vi "Dashboard Main.vi"() -> ()   [LabVIEW 2018]
uses:
  <vilib>/Utility/miscctls.llb/LVRowAndColumnTypeDef.ctl
  <vilib>/event_ctls.llb/eventvkey.ctl
  <vilib>/Utility/xml.llb/Read From XML File(array).vi
  <vilib>/Utility/xml.llb/Write to XML File(string).vi
  <vilib>/Rock Robotics/Network Tables/NT Read Boolean.vi
  <vilib>/Rock Robotics/Network Tables/NT Write Boolean.vi
  <vilib>/Rock Robotics/WPI/Dashboard/WPI_DashboardLogging Global.vi
  <vilib>/vision/NI_Vision_Development_Module.lvlib
panel:
  in  "TCP":refnum<k5>
  in  "Rec Mode":enum32{"Stop", "Record", "Playback"}(radio)
  out "Image Message":string="Timeout in Camera Communications"
  in  "Dashboard Tab":T1(tab)=enum."TeleOp"
  in  "CheckList":i32(listbox)
  in  "Driver Profile":u16(ring) items=["N/A"]
  in  "Camera Name":string(combo)="limelight"
  in  "Camera Settings":T2={"Frame Rate"=20, "Compression"=60, "Size"=1, "DB Camera Config"=FALSE} {"Size" items=["640x480", "320x240", "160x120"]}
  in  "Warning Time (s)":dbl=30.0
  in  "Autonomous Play":u16(ring) items=["N/A"]
  in  "Refresh_Auto_Play_List":bool
  out "Pressure_Leak":bool
  out "Ret_CARGO Right":bool
  out "Ret_HATCH Right":bool
  out "Ret_CARGO Left":bool
  out "Ret_HATCH Left":bool
  out "Ret_CARGO Center":bool
  out "Elevator_Motor_Failure_2":bool
  out "Elevator_Stall":bool
  out "Range_Color_Front-Right":u32(colorbox)
  in  "Right":bool
  in  "Reticule":T3(ring)
  in  "Save":bool
  in  "Up":bool
  in  "Down":bool
  in  "Left":bool
  out "Out_Of_Time":bool caption="Mode_Butterfly"
  out "Match Time(s)":sgl
  out "Intake_In":bool caption="Mode_Butterfly"
  in  "Climb_Safety":bool
  out "Master_Caution":bool caption="Mode_Butterfly"
  out "Climb_Sequence":string
  out "Range_to_Target (R)":i16(slide)=-100 scale=-10.0..-50.0
  out "Range_to_Target (L)":i16(slide)=-100 scale=-50.0..-10.0
  out "Tilt_Interlock":bool
  out "Battery_Critical":bool
  out "Battery_Voltage":dbl(slide) scale=11.0..13.0
  out "COM_Warning":bool
  out "Elevator_Moving":bool caption="Mode_Butterfly"
  out "Range_Color_Back":u32(colorbox)
  out "Range_Color_Front-Left":u32(colorbox)
  out "Range_Color_Right":u32(colorbox)
  out "Range_Color_Left":u32(colorbox)
  out "Hatch_Ship_Light":bool
  out "Hatch_Rocket_1_Light":bool
  out "Hatch_Ground_Light":bool
  out "Hatch_Feeder_Light":bool
  out "Hatch_Rocket_2_Light":bool
  out "Hatch_Rocket_3_Light":bool
  out "Pressure_Visualize":dbl(slide) scale=0.0..120.0
  out "Autopilot":bool caption="Mode_Butterfly"
  in  "Master_Safety_Override_1":bool
  in  "Master_Safety_Override_2":bool
  out "Climb_Light":bool
  out "At Climb_Height":bool caption="Mode_Butterfly"
  out "PTO_Engaged":bool caption="Mode_Butterfly"
  in  "Climb":bool
  out "Mode_Butterfly":bool
  out "Compressor_On":bool
  out "Hatch_Ejection_State":bool caption="Mode_Butterfly"
  out "Elevator_Brake_State":bool
  out "Mode_Shift":bool caption="Mode_Butterfly"
  out "Capture_Cargo":bool caption="Mode_Butterfly"
  out "Capture_Hatch":bool caption="Mode_Butterfly"
  in  "Hatch_Ground":bool
  in  "Hatch_Feeder":bool
  in  "Hatch_Rocket_2":bool
  in  "Hatch_Rocket_1":bool
  in  "Hatch_Ship":bool
  in  "Hatch_Rocket_3":bool
  out "Elevator_Stow_Light":bool
  in  "Elevator_Stow":bool
  out "Cargo_Ground_Light":bool
  out "Cargo_Feeder_Light":bool
  out "Cargo_Ship_Light":bool
  out "Cargo_Rocket_3_Light":bool
  in  "Cargo_Ground":bool
  in  "Cargo_Feeder":bool
  out "Cargo_Rocket_2_Light":bool
  out "Cargo_Rocket_1_Light":bool
  in  "Cargo_Ship":bool
  in  "Cargo_Rocket_1":bool
  in  "Cargo_Rocket_2":bool
  in  "Cargo_Rocket_3":bool
  out "State_Conflict":bool caption="Mode_Butterfly"
  out "Combined Camera Feed":T4(plugin-control)
  out "Elevator_Pos_Visual":dbl(slide) scale=34.5..89.0
  in  "Vision_Target_L_R":bool
  out "Elevator_Goal_Visual":dbl(slide) scale=34.5..89.0
  out "Elevator_Power":dbl(knob) scale=-1.0..1.0
  in  "Climb_Level":u8(slide)=1 scale=0.0..2.0
  out "E1 Warning":bool
  out "E2 Warning":bool
  out "E3 Warning":bool
  out "Elevator_3_Current":dbl format="%.1g"
  out "Elevator_2_Current":dbl format="%.1g"
  out "Elevator_1_Current":dbl format="%.1g"
  out "Slow_Loop":bool
  in  "Elevator_Kf_1":dbl(slide)=0.2 min=0.0 max=1.0 scale=0.0..1.0
  in  "Elevator_Kf_2":dbl(slide)=0.2 min=0.0 max=1.0 scale=0.0..1.0
  in  "Elevator_Kf_3":dbl(slide) min=0.0 max=1.0 scale=0.0..1.0
  in  "Select Auto":string(combo)="Select Autonomous ..."
  out "Camera Perf":string
  in  "Elevator_Kf_Climb":dbl(slide)=0.1 min=0.0 max=1.0 scale=0.0..1.0
  out "Control Loop Time (ms)":u32
  in  "Vacuum_Pump":dbl(slide)=0.6 min=0.0 max=1.0 scale=0.0..1.0
  out "Range_Right":dbl format="%.1g"
  in  "Elevator_Manual":bool
  in  "Drive_Encoder_Reset":bool
  out "Right_Drive_Pos":dbl
  out "Left_Drive_Pos":dbl
  out "Range_Left":dbl format="%.1g"
  out "Range_Front-Left":dbl format="%.1g"
  out "Range_Front-Right":dbl format="%.1g"
  out "Left_Drive_Vel":dbl format="%.1g"
  out "Right_Drive_Vel":dbl format="%.1g"
  out "Elevator_Pos":dbl format="%.1g"
  out "Range_Back":dbl
  out "Tank_Pressure":dbl format="%.1f"
  in  "Super_Test_Mode":bool
  out "Ground_Height":dbl format="%.1g"
  in  "Overclock":bool=TRUE
  in  "Reinit_Stow_Vacuum":bool
  in  "LimeLight_Override":bool
  out "Elevator_Encoder_Malfunction":bool
  out "Elevator_Motor_Failure":bool
  out "Robot_On_Ground":bool=TRUE
  out "Robot_Off_Ground":bool
  out "Check_Limit_Switch":bool
  in  "Tilt_Safety_Override":bool
  in  "Defense_Driving":bool
  out "Combined Error String":string
  out "NT Connection":bool
  out "Mode":T5(ring)=enum."Auto Disabled"
  in  "Test Slider":dbl(slide) scale=0.0..100.0 scale format="%#_3g"
  in  "On/Off":bool caption="Solenoid"
  in  "Test Name":u16(ring) items=["Select the test to run..."]
  in  "Test Tree":string(tree)
  in  "Motor":cluster{"Value":dbl, "Enable":bool} {"Value" scale=-1.0..1.0 scale format="%#_3g"}
  out "Progress":T6 {"Test Progress" scale=0.0..100.0}
  in  "Rev/Fwd":cluster{"Forward":bool, "Reverse":bool}
  in  "Test Ring":u16(ring) items=["Monochrome", "Color"]
  out "Cmd Status":string
  in  "Execute Command":bool
  in  "Command Params":string[][](table)
  in  "Command Selection":i32(listbox)
  out "Tree":string(tree)
  out "Background":bool
  # "Refresh Auto Plays List"
  # "Camera Selection"
  # "Match End Warning (s)"
  # "Camera Settings"
  # "Safe"
  # "89.0"
  # "11"
  # "13"
  # "120"
  # "0"
  # "Valkyrie"
  # "B"
  # "3"
  # "2"
  # "0"
  # "34.5"
  # "Control Loop (ms)"
  # "Elevator Feed Forward Coefficients"
  # "Drive Wheel Velocities (ft/s)"
  # "Manual Elevator Override"
  # "Tilt Interlock Off"
  # "Wide-Cam Override"
  # "Reinit.  Vacuum in Stow"
  # "Super Test Mode"
  # "Elevator Position (in)"
  # "Prox Sensors (in)"
  # "Auto Elevator"
  # "Safe"
  # "Vacuum \nPump Power"
  # "Normal"
  # "Normal"
  # "Safe"
  # "Stage 2"
  # "Stage 3"
  # "Climb"
  # "Ground Height (in)"
  # "Elevator Motor Currents (A)"
  # "On \nGround"
  # "Off\nGround"
  # "E1"
  # "E2"
  # "E3"
  # "Tank Pressure (psi)"
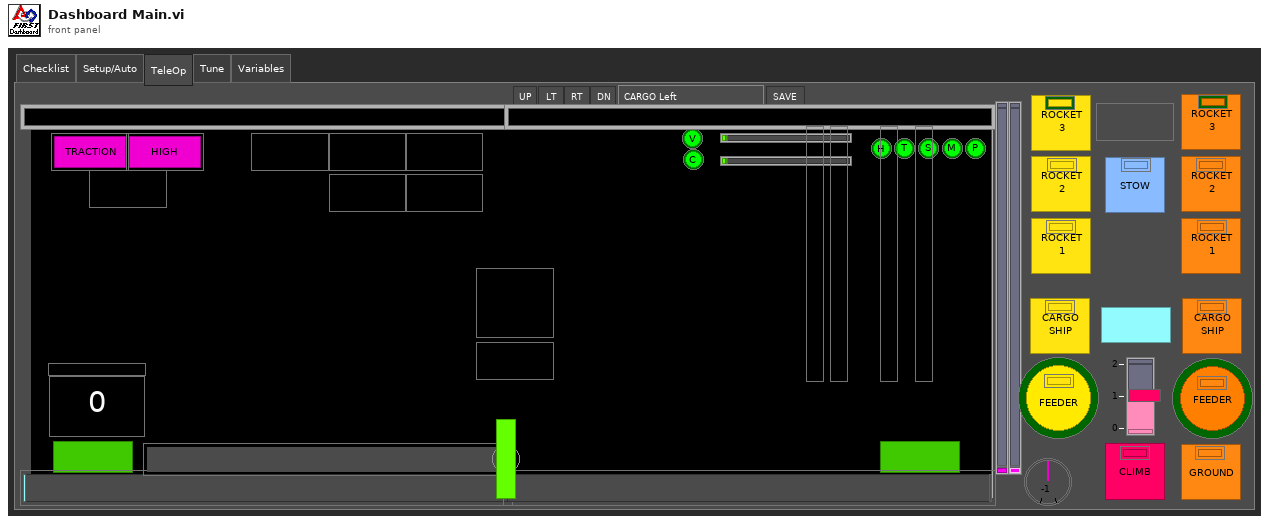
[diagram p1: front panel]
types:
  T1 = enum32{"Checklist", "Setup/Auto", "TeleOp", "Tune", "NT", "Test", "Commands", "Variables"}
  T2 = cluster{"Frame Rate":i32, "Compression":i32, "Size":u16, "DB Camera Config":bool}
  T3 = enum16{"CARGO Left", "CARGO Right", "HATCH Left", "HATCH Right", "CARGO Center"}
  T4 = typedef "IMAQ Image.ctl" = refnum<image>
  T5 = enum8{"Tele-Op Disabled", "Tele-Op Enabled", "Auto Disabled", "Auto Enabled", "Test Disabled", "Test Enabled", "Disconnected", "No Code", "E-Stop"}
  T6 = cluster{"Test Progress":u8, "Test Progress Text":string}
  T7 = cluster{"Save Path":path, "Interval (s)":dbl, "Keep":i32}
  T8 = enum32{"Drive", "Camera", "Basic", "Custom", "Test", "Commands", "Checklist", "Variables"}
  T9 = cluster{"IDs":cluster{"RPC field ID":u16, "Unique ID":u16}, "String":string}
  T10 = typedef "Image Type" = u32
  T11 = cluster{"Camera Name":string, string, "Saved DB Images Info":cluster{"Save Path":path, "Interval (s)":dbl, "Keep":i32}}
  T12 = cluster{"Ret_CARGO Left":refnum<vi>, "Ret_CARGO Right":refnum<vi>, "Ret_HATCH Left":refnum<vi>, "Ret_HATCH Right":refnum<vi>, "Ret_CARGO Center":refnum<vi>}
  T13 = enum32{"Checklist", "-", "TeleOp", "Tune", "NT", "Test", "Commands", "Variables"}
  T14 = cluster{"Error Strings":string, "Disable Counts":cluster{u16, u16}, "Rail Faults":cluster{u16, u16, u16}, "Robot IP":string, "DB Mode":u8, "Event Info":cluster{"Name":string, "Type":u8, "Number":u16, "Replay":u8}}
  T15 = cluster{"Storage":cluster{"Disk Free":u64, "RAM Block":u32, "RAM free":u32}, "CPU Utilization":cluster{"CPU % ISR":sgl, "CPU % Time Crit":sgl, "CPU % Timed Str":sgl, "CPU % High":sgl, "CPU % Above":sgl, "CPU % Normal":sgl, "CPU % Low":sgl}, "CAN":cluster{"% Bus Utilization":sgl, "Bus Off Cnt":u32, "TX_FIFO Full Cnt":u32, "Receive Error Cnt":u8, "Transmit Error Cnt":u8}, "HID":cluster{"HID Outputs":u32, "Rumble Low":u16, "Rumble High":u16}[]}
  T16 = cluster{"Status bits":cluster{"Test Mode":bool, "Autonomous":bool, "Enabled":bool, "Code Start":bool, "Brownout":bool, "Reserved 2":bool, "Reserved 3":bool, "E-Stop":bool}, "Code Trace":cluster{"Disabled":bool, "TeleOp":bool, "Auto":bool, "Test":bool}, "Controller Type":enum16{"unknown", "cRIO", "roboRio"}, "Code?":enum16{"unknown", "noCode", "code"}, "Battery V":dbl}
  T17 = cluster{"Control Bits":cluster{"TestMode":bool, "Autonomous":bool, "Enabled":bool, "FMS Present":bool, bool, bool, bool, "E-Stop":bool}, "Team Station ":u8, "Countdown":sgl, "Joystick Values":cluster{"Axes":dbl[], "Buttons":bool[], "POVs":i16[]}[]}
  T18 = cluster{"Operation":enum16{"Update", "Clear"}, "Color Box":u32}[]
  T19 = typedef "eventvkey.ctl" = enum16{"ASCII", "Enter", "Return", "Shift", "Ctrl", "Alt", "Cmd", "Opt", "Caps", "NumLock", "Clear", "Break", "Up", "Down", "Left", "Right", "Insert", "Delete", "Home", "End", "PageUp", "PageDown", "Escape", "Help", "Pause", "ScrollLock", "F1", "F2", "F3", "F4", "F5", "F6", "F7", "F8", "F9", "F10", "F11", "F12", "F13", "F14", "F15", "F16", "F17", "F18", "F19", "F20", "F21", "F22", "F23", "F24", "Play", "VolumeUp", "VolumeDown", "Mute", "Two Byte Char"}
  T20 = cluster{"Image Size":bool, "Image Type":bool, "Pixel Value":bool, "ROI Information":bool, "Zoom Factor":bool}
  T21 = cluster{"Operation":enum16{"Update", "Clear"}, "Color Box":u32}
  T22 = typedef "LVRowAndColumnTypeDef.ctl" = cluster{"Row":i32, "Column":i32}
  T23 = cluster{"Shift":bool, "Ctrl":bool, "Alt":bool, "Cmd":bool, "Opt":bool}
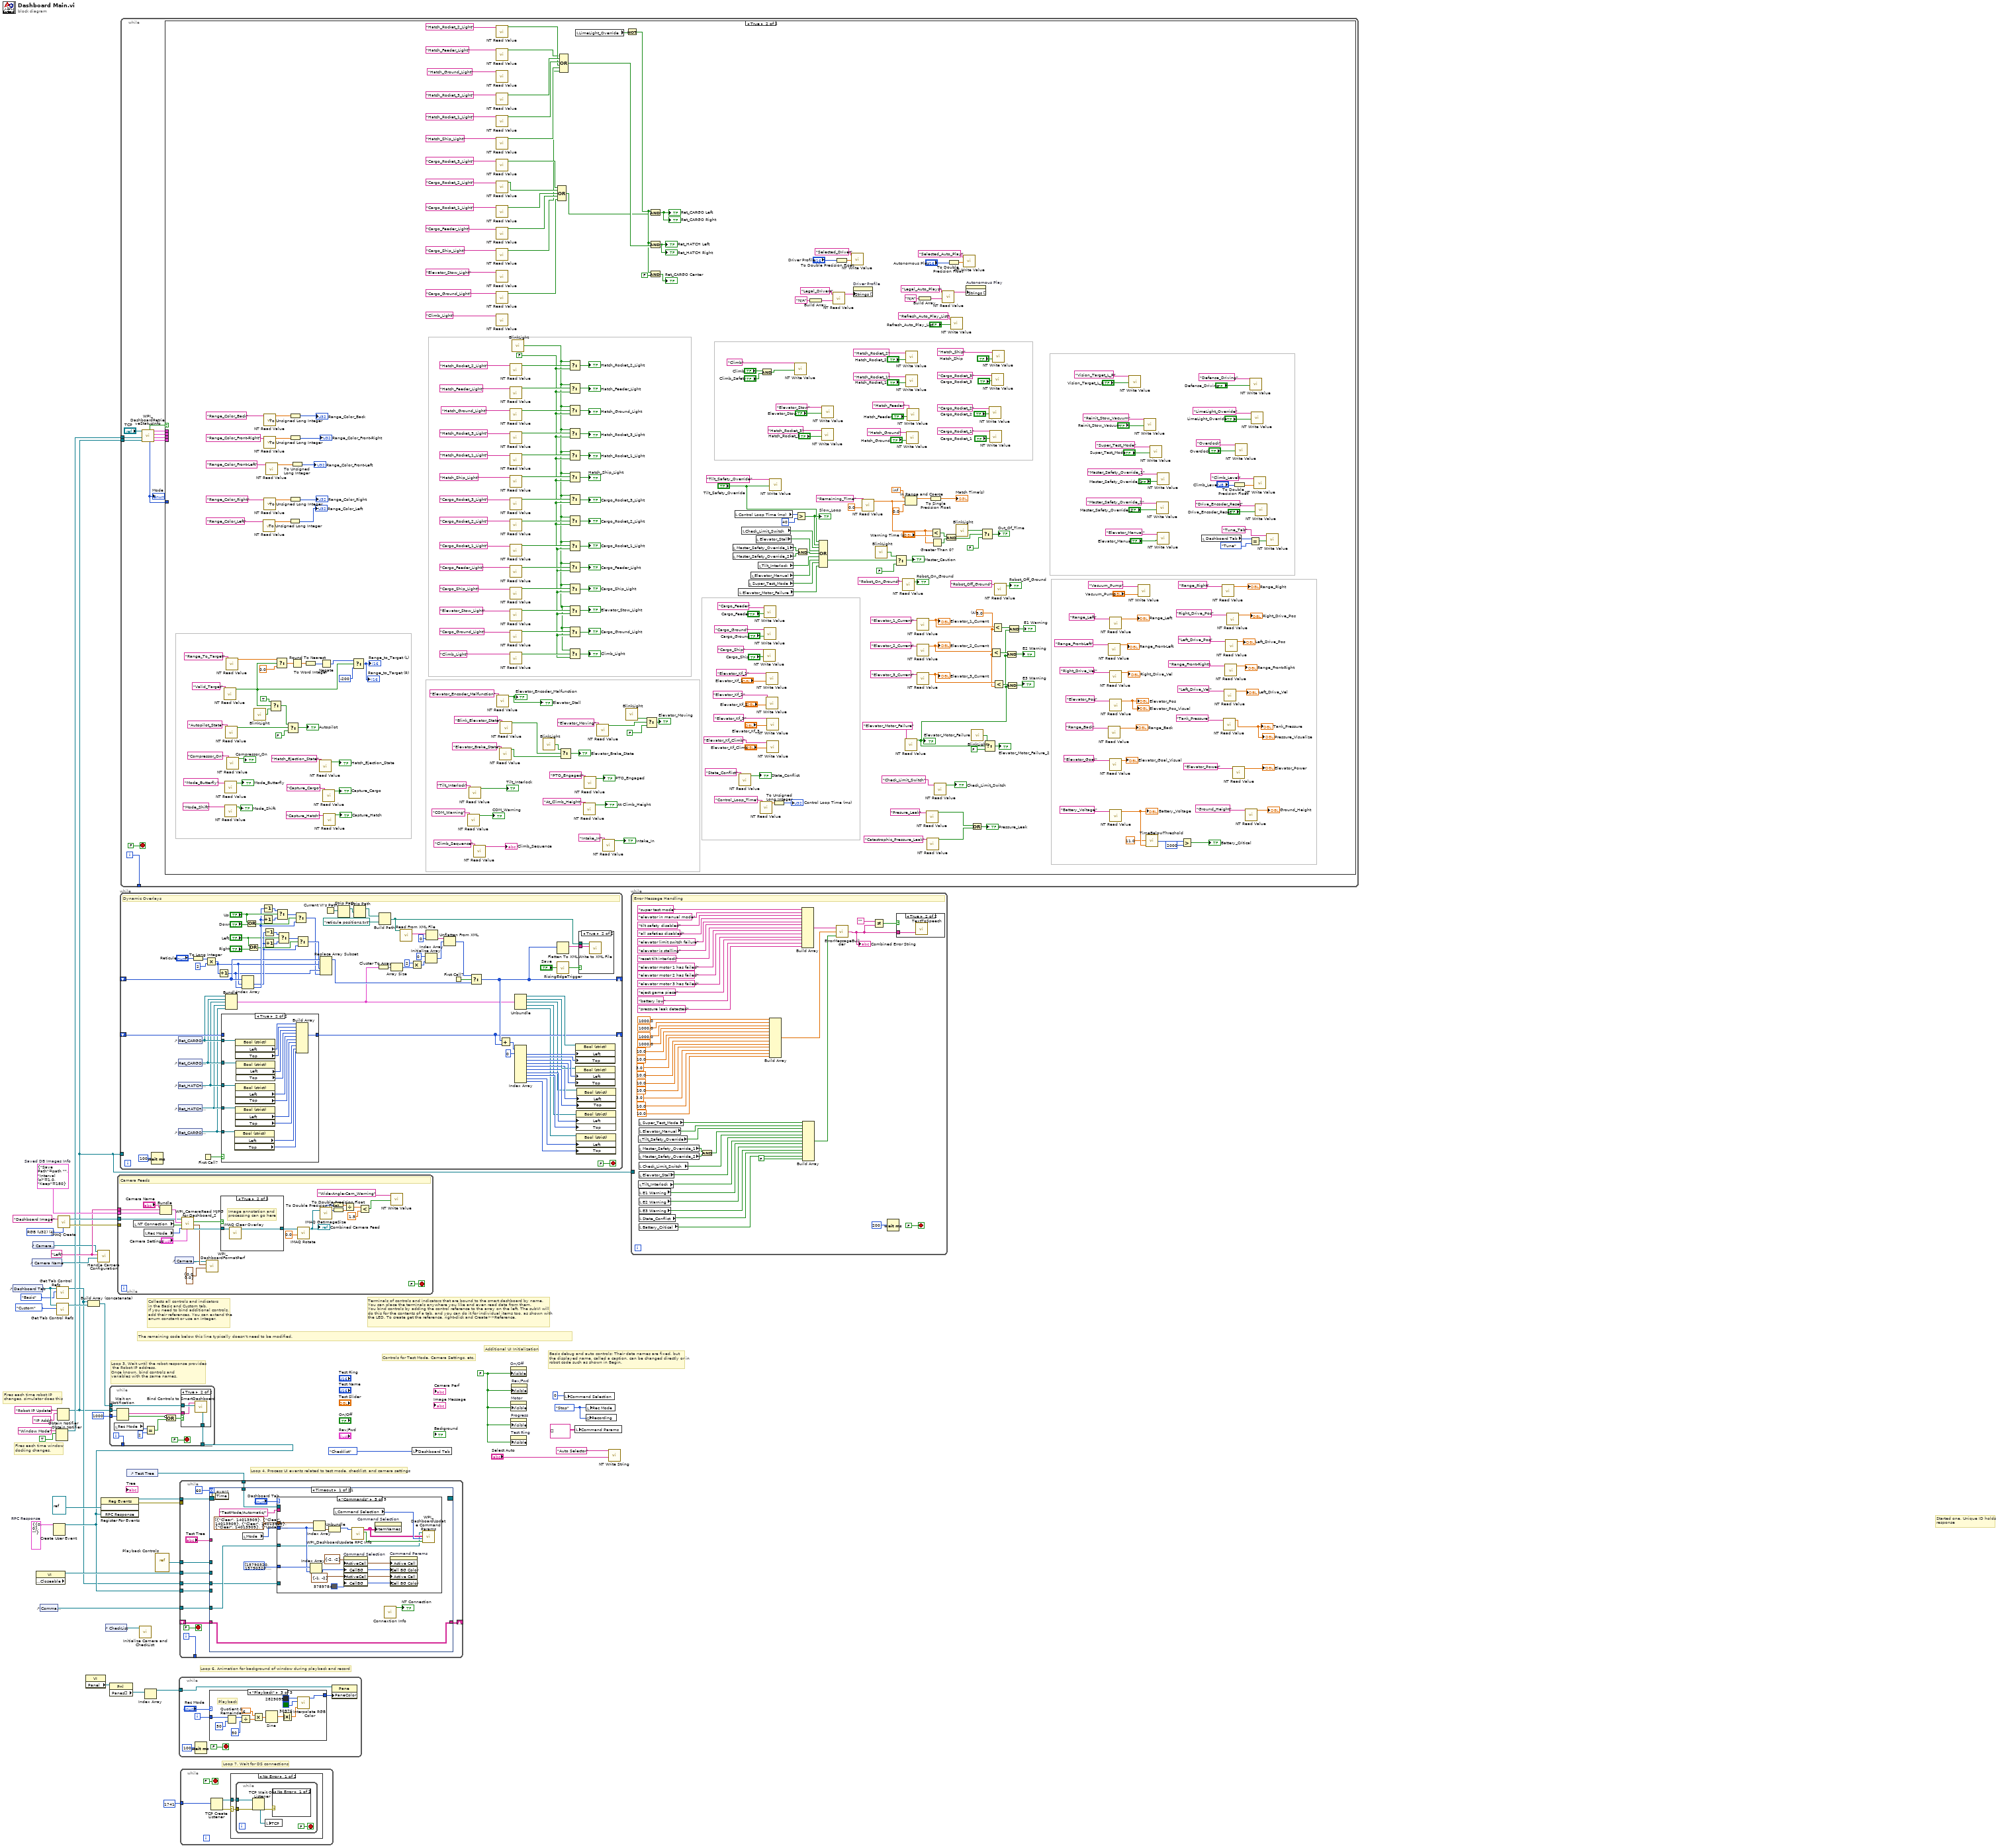
[diagram p0: block diagram]
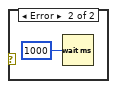
[diagram p5: hidden frame]
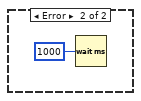
[diagram p6: hidden frame]
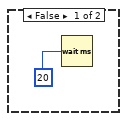
[diagram p7: hidden frame]
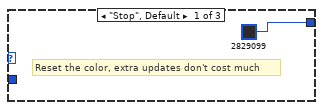
[diagram p8: hidden frame]
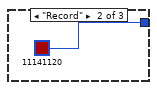
[diagram p9: hidden frame]
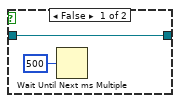
[diagram p11: hidden frame]
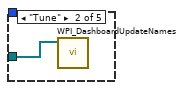
[diagram p13: hidden frame]
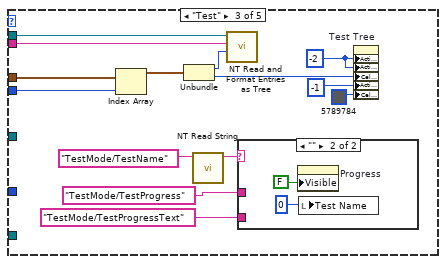
[diagram p14: hidden frame]
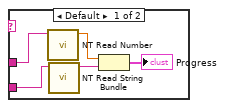
[diagram p15: hidden frame]
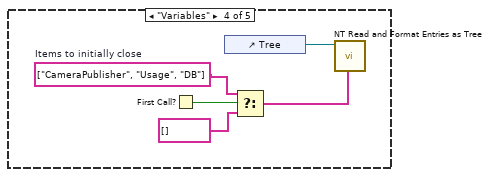
[diagram p16: hidden frame]
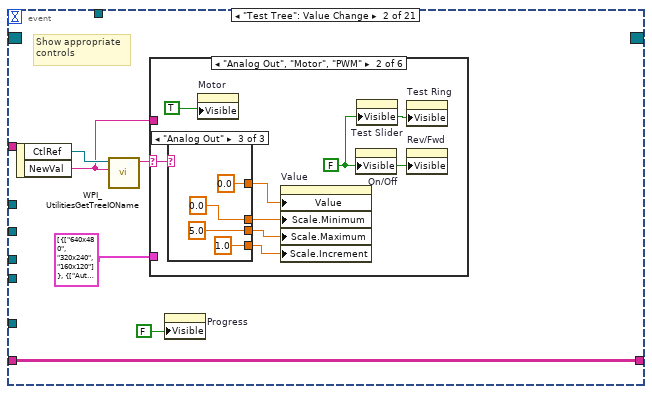
[diagram p17: hidden frame]
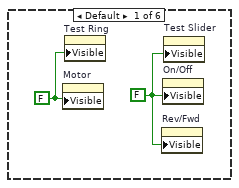
[diagram p18: hidden frame]
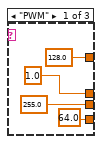
[diagram p19: hidden frame]
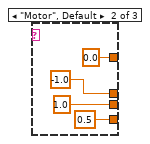
[diagram p20: hidden frame]
diagram:
  w4 = T7 {"Save Path"=path "", "Interval (s)"=1.0, "Keep"=180}  # Saved DB Images Info
  w3 = "Left"
  w15 = T9 {"IDs"={"RPC field ID"=0, "Unique ID"=0}, "String"=""}  # RPC Response
  w25 = enum32{"Stop", "Record", "Playback"}."Stop" ("Rec Mode")
  w19 = FALSE ("Visible")
  w42 = T10 4 items=["Grayscale (U8)", "Grayscale (I16)", "Grayscale (SGL)", "Complex (CSG)", "RGB (U32)", "HSL (U32)", "RGB (U64)"] ("Image Type")
  # "Started one, Unique ID holds\nresponse"
  # "Loop 7. Wait for DS connections"
  # "Basic debug and auto controls: Their data names are fixed, but\nthe displayed name, called a caption, can be changed directly or in\nrobot code such as shown in Begin."
  # "Controls for Test Mode, Camera Settings, etc."
  # "Additional UI Initialization"
  # "Loop 6. Animation for background of window during playback and record"
  # "Fires each time robot IP\nchanges, simulator does this"
  # "Fires each time window\ndocking changes."
  # "Collects all controls and indicators\nin the Basic and Custom tab.\nIf you need to bind additional controls,\nadd their references. You can extend the\nenum constant or use an integer."
  # "The remaining code below this line typically doesn't need to be modified."
  # "Loop 4. Process UI events related to test mode, checklist, and camera settings"
  # "Terminals of controls and indicators that are bound to the smart dashboard by name.\nYou can place the terminals anywhere you like and even read data from them.\nYou bind controls by adding the control reference to the array on the left. The subVI will\ndo this for the contents of a tab, and you can do it for individual items too, as shown with\nthe LED. To create get the reference, right-click and Create>>Reference."
  # "Loop 3. Wait until the robot response provides\n the Robot IP address.\nOnce known, bind controls and\nvariables with the same names."
  n1 = control-ref of="Dashboard Tab"() -> (w23:refnum<vi>)
  n2 = control-ref of="Camera Name"() -> (w10:refnum<vi>)
  n3 = control-ref of="Camera Settings"() -> (w2:refnum<vi>)
  n4 = property class="VI" props=["Front Panel.Closeable"]() -> (reference out=w24:refnum<vi>)  [unwired: 2 in, 2 out]
  n5 = control-ref of="Command Params"() -> (w11:refnum<vi>)
  n6 = Create User Event(user event datatype=w15) -> (user event=w12:refnum<user-event>)  [unwired: 1 in, 1 out]
  n7 = Obtain Notifier(name (unnamed)="Window Mode", notification data type=TRUE) -> (notifier out=w18:refnum<notifier>)  [unwired: 2 in, 2 out]
  n8 = call <vilib>:"Get Tab Control Refs.vi"("Page Index"=T8."Basic" ("Dashboard Tab"), "TabControl in"=w23) -> ("ControlsOnPage"=w9:refnum<vi>[])  [unwired: 9 in]
  n9 = call <vilib>:"Get Tab Control Refs.vi"("Page Index"=T8."Custom" ("Dashboard Tab"), "TabControl in"=w23) -> ("ControlsOnPage"=w22:refnum<vi>[])  [unwired: 9 in]
  n10 = Obtain Notifier(name (unnamed)="Robot IP Update", notification data type="IP Addr" ("name (unnamed)")) -> (notifier out=w1:refnum<notifier>)  [unwired: 2 in, 2 out]
  n11 = call "IMAQ Create"("Image Name"="Dashboard Image", "Image Type"=w42) -> ("New Image"=w40:T4, "error out"=w39:errorcluster)  [unwired: 2 in, 1 out]
  n12 = property class="VI"() -> ("Panel"=w32:refnum<vi>)  [unwired: 2 in, 2 out]
  n13 = Build Array (concatenate)(w9, w22) -> (w21:refnum<vi>[])
  n14 = call "Handle Camera Configuration.vi"("CameraNameRef"=w10, "Display Name"=w3, "ClusterRef"=w2) -> ()  [unwired: 9 in]
  n15 = register-events(refnum<vi> refnum, w12) -> (reference out=w29:refnum<event-registration>, error out=w28:errorcluster)  [unwired: 2 in]
  n16 = control-ref of="CheckList"() -> (w20:refnum<vi>)
  n17 = while {
    tunnel: w21 -> [w54]
    tunnel: w1 -> [w52]
    tunnel: [w50] -> _
    tunnel: u32 1000 ("milliseconds to wait") -> [w49]
    tunnel: w12 -> [w43]
    i -> [w50]
    stop <- FALSE stop-if-true
    n18 = local read "Rec Mode"() -> (w45:enum32{"Stop", "Record", "Playback"})
    n19 = Wait on Notification(notifier=w52, timeout in ms (-1)=w49) -> (notification=w51:string, timed out?=w47:bool)  [unwired: 2 in, 2 out]
    n20 = Equal?(x=w45, y=u16 2 ("Rec Mode")) -> (x = y?=w46:bool)
    n21 = Compound Arithmetic op=OR(invert w47, w46) -> (w48:bool)
    n22 = case shown="True" w48 {
      tunnel: w54 -> [_ w57]
      tunnel: w51 -> [_ w56]
      tunnel: w43 -> [_ w55]
      frame False {
      }
      frame True {
        n23 = call <vilib>:"Bind Controls to SmartDashboard.vi"("RPC ref"=w55, "Bound Control Refs"=w57, "Server IP Address"=w56) -> ()  [unwired: 9 in]
      }
    }
  }
  n24 = property class="Pnl"(reference=w32) -> ("Panes[]"=w33:refnum<vi>[])  [unwired: 1 in, 2 out]
  n25 = while {
    tunnel: w40 -> [w72]
    tunnel: w39 -> [_]
    tunnel: w4 -> [w77]
    tunnel: w3 -> [w75]
    stop <- FALSE stop-if-true
    # "Camera Feeds"
    n26 = local read "NT Connection"() -> (w78:bool)
    n27 = local read "Rec Mode"() -> (w79:enum32{"Stop", "Record", "Playback"})
    n28 = Bundle("Camera Name"="Camera Name", w75, "Saved DB Images Info"=w77) -> (w76:T11)  [unwired: 1 in]
    n29 = control-ref of="Camera Perf"() -> (w73:refnum<vi>)
    n30 = call <vilib>:"WPI_CameraRead MJPG for Dashboard_2.vi"("Camera Settings"="Camera Settings", "Rec Mode"=w79, "NT Connection"=w78, "Capture Info"=w76, "Image in"=w72) -> ("perf info"=w74:cluster{"Bandwidth (Mbps)":dbl, "fps":dbl}, "Active"=w80:bool, "Image\\ out"=w81:T4)  [unwired: 4 in]
    n31 = call <vilib>:"WPI_DashboardFormatPerf.vi"("Right Camera Perf"=cluster{"Bandwidth (Mbps)":dbl, "FPS":dbl} {"Bandwidth (Mbps)"=0.0, "FPS"=0.0}, "Performance"=w74, "String in"=w73) -> ()  [unwired: 9 in]
    n32 = case shown="True" w80 {
      tunnel: w81 -> [w83 w86]
      tunnel: [w83 w85] -> w71
      frame False {
        n33 = Wait Until Next ms Multiple(millisecond multiple=u32 500) -> ()  [unwired: 1 out]
      }
      frame True {
        # "Image annotation and\nprocessing can go here"
        n34 = call "IMAQ Clear Overlay"("Image"=w86) -> ("Image Out"=w85:T4)  [unwired: 2 in, 8 out]
      }
    }
    n35 = call "IMAQ Rotate"("Angle (degrees)"=sgl 0.0, "Image Src"=w71) -> ("Image Dst Out"=w68:T4)  [unwired: 8 in, 1 out]
    "Combined Camera Feed" <- w68
    n36 = call "IMAQ GetImageSize"("Image"=w68) -> ("Y Resolution"=w64:i32, "X Resolution"=w65:i32)  [unwired: 3 in, 1 out]
    n37 = To Double Precision Float(number=w65) -> (double precision float=w67:dbl)
    n38 = To Double Precision Float(number=w64) -> (double precision float=w66:dbl)
    n39 = Divide(x=w67, y=w66) -> (x/y=w63:dbl)
    n40 = Less?(x=w63, y=1.5) -> (x < y?=w61:bool)
    n41 = call-poly <vilib>:"NT Write Value.vi"("Boolean"=w61, "Name"="Wide-Angle-Cam_Warning") -> ()  [unwired: 9 in, 1 out]
  }
  n42 = while {
    shift-right: [w102] -> _
    shift-left: _ -> [w155]
    shift-right: [w106] -> _
    shift-left: _ -> [w145]
    tunnel: w1 -> [_]
    stop <- FALSE stop-if-true
    # "Dynamic Overlays"
    n43 = Wait (ms)(milliseconds to wait=u32 100) -> ()  [unwired: 1 out]
    n44 = control-ref of="Ret_CARGO Left"() -> (w111:refnum<vi>)
    n45 = control-ref of="Ret_CARGO Right"() -> (w110:refnum<vi>)
    n46 = control-ref of="Ret_HATCH Left"() -> (w96:refnum<vi>)
    n47 = control-ref of="Ret_HATCH Right"() -> (w95:refnum<vi>)
    n48 = control-ref of="Ret_CARGO Center"() -> (w92:refnum<vi>)
    n49 = To Long Integer(number="Reticule") -> (32bit integer=w136:i32)
    n50 = First Call?() -> (First Call?: T/F=w119:bool)
    n51 = Multiply(x=w136, y=2) -> (x*y=w135:i32)
    n52 = Increment(x=w135) -> (x+1=w114:i32)
    n53 = case shown="True" w119 {
      tunnel: w111 -> [_ w176]
      tunnel: [w160 w173] -> w102
      tunnel: w155 -> [w160 _]
      tunnel: w110 -> [_ w170]
      tunnel: w96 -> [_ w169]
      tunnel: w95 -> [_ w168]
      tunnel: w92 -> [_ w163]
      frame False {
      }
      frame True {
        n54 = property class="Bool (strict)"(reference=w163) -> ("Left"=w162:i32, "Top"=w161:i32)  [unwired: 1 in, 2 out]
        n55 = property class="Bool (strict)"(reference=w176) -> ("Left"=w175:i32, "Top"=w174:i32)  [unwired: 1 in, 2 out]
        n56 = property class="Bool (strict)"(reference=w169) -> ("Left"=w167:i32, "Top"=w166:i32)  [unwired: 1 in, 2 out]
        n57 = property class="Bool (strict)"(reference=w168) -> ("Left"=w165:i32, "Top"=w164:i32)  [unwired: 1 in, 2 out]
        n58 = property class="Bool (strict)"(reference=w170) -> ("Left"=w172:i32, "Top"=w171:i32)  [unwired: 1 in, 2 out]
        n59 = Build Array(w175, w174, w172, w171, w167, w166, w165, w164, w162, w161) -> (w173:i32[])
      }
    }
    n60 = Bundle("Ret_CARGO Left"=w111, "Ret_CARGO Right"=w110, "Ret_HATCH Left"=w96, "Ret_HATCH Right"=w95, "Ret_CARGO Center"=w92) -> (w104:T12)  [unwired: 1 in]
    n61 = Index Array(array=w145, index #1=w135, index #2=w114) -> (element #1=w139:i32, element #2=w147:i32)
    n62 = Or(x="Up", y="Down") -> (x .or. y?=w151:bool)
    n63 = Or(x="Left", y="Right") -> (x .or. y?=w141:bool)
    n64 = Decrement(x=w147) -> (x-1=w154:i32)
    n65 = Increment(x=w147) -> (x+1=w153:i32)
    n66 = Decrement(x=w139) -> (x-1=w144:i32)
    n67 = Increment(x=w139) -> (x+1=w143:i32)
    n68 = Select(t=w154, s="Up", f=w153) -> (s? t:f=w152:i32)
    n69 = Select(t=w144, s="Left", f=w143) -> (s? t:f=w142:i32)
    n70 = Select(t=w152, s=w151, f=w147) -> (s? t:f=w113:i32)
    n71 = Select(t=w142, s=w141, f=w139) -> (s? t:f=w140:i32)
    n72 = Replace Array Subset(array=w145, new element #1=w140, index #1=w135, new element #2=w113, index #2=w114) -> (w112:i32[])
    n73 = Current VI's Path() -> (path=w127:path)
    n74 = Strip Path(path=w127) -> (stripped path=w126:path)  [unwired: 1 out]
    n75 = Strip Path(path=w126) -> (stripped path=w125:path)  [unwired: 1 out]
    n76 = Cluster To Array(cluster=w104) -> (array=w109:refnum<vi>[])
    n77 = Build Path(base path=w125, name or relative path=path "reticule positions.txt" ("XML File Path")) -> (appended path=w124:path)
    n78 = Array Size(array=w109) -> (size(s)=w105:i32)
    n79 = call-poly <vilib>:"Read From XML File.vi"("XML File Path"=w124) -> ("XML Elements"=w123:string[])  [unwired: 8 in, 2 out]
    n80 = Multiply(x=2 ("dimension size"), y=w105) -> (x*y=w118:i32)
    n81 = Initialize Array(0, w118) -> (w88:i32[])
    n82 = Index Array(array=w123, index=0) -> (element=w121:string)
    n83 = Unflatten From XML(xml string=w121, type=w88) -> (value=w87:i32[])  [unwired: 1 in, 1 out]
    n84 = First Call?() -> (First Call?: T/F=w146:bool)
    n85 = Select(t=w87, s=w146, f=w112) -> (s? t:f=w106:i32[])
    n86 = Add(x=w106, y=w102) -> (x+y=w103:i32[])
    n87 = Unbundle(w104) -> ("Ret_CARGO Left"=w108:refnum<vi>, "Ret_CARGO Right"=w107:refnum<vi>, "Ret_HATCH Left"=w94:refnum<vi>, "Ret_HATCH Right"=w93:refnum<vi>, "Ret_CARGO Center"=w91:refnum<vi>)
    n88 = Index Array(array=w103, index #1=0 ("index")) -> (element #1=w133:i32, element #2=w132:i32, element #3=w116:i32, element #4=w115:i32, element #5=w100:i32, element #6=w99:i32, element #7=w98:i32, element #8=w97:i32, element #9=w90:i32, element #10=w89:i32)  [unwired: 9 in]
    n89 = Flatten To XML(anything=w106) -> (xml string=w131:string)
    n90 = call "RisingEdgeTrigger.vi"("Raw Signal"="Save") -> ("Trigger"=w130:bool)
    n91 = property class="Bool (strict)"(reference=w108, "Left"=w133, "Top"=w132) -> ()  [unwired: 1 in, 2 out]
    n92 = property class="Bool (strict)"(reference=w107, "Left"=w116, "Top"=w115) -> ()  [unwired: 1 in, 2 out]
    n93 = property class="Bool (strict)"(reference=w93, "Left"=w98, "Top"=w97) -> ()  [unwired: 1 in, 2 out]
    n94 = property class="Bool (strict)"(reference=w91, "Left"=w90, "Top"=w89) -> ()  [unwired: 1 in, 2 out]
    n95 = property class="Bool (strict)"(reference=w94, "Left"=w100, "Top"=w99) -> ()  [unwired: 1 in, 2 out]
    n96 = case shown="True" w130 {
      tunnel: w131 -> [_ w159]
      tunnel: w124 -> [_ w158]
      frame False {
      }
      frame True {
        n97 = call-poly <vilib>:"Write to XML File.vi"("XML Input"=w159, "XML File Path"=w158) -> ()  [unwired: 7 in, 3 out]
      }
    }
  }
  n98 = while {
    tunnel: [w186] -> _
    tunnel: w1 -> [w180]
    tunnel: w18 -> [w177]
    i -> [w186]
    stop <- FALSE stop-if-true
    n99 = call <vilib>:"WPI_DashboardRetrieveStatusInfo.vi"("Binding Refnum"=w180, "Window Mode Notifier"=w177, "TCP Cnx"="TCP") -> ("Power and Errors"=w181:T14, "Robot Metrics"=w184:T15, "Status Info"=w185:T16, "Control Info"=w182:T17, "Robot Mode"=w179:T5, "Process?"=w183:bool)  [unwired: 3 in]
    "Mode" <- w179
    n100 = case shown="True" w183 {
      tunnel: w185 -> [_ _]
      tunnel: w184 -> [_ _]
      tunnel: w182 -> [_ _]
      tunnel: w181 -> [_ _]
      tunnel: w179 -> [_ _]
      frame False {
        n101 = Wait (ms)(milliseconds to wait=u32 20) -> ()  [unwired: 1 out]
      }
      frame True {
        w229 = 5.0  # (A)
        w374 = FALSE ("f")
        n102 = call-poly <vilib>:"NT Read Value.vi"("Name"="Valid_Target") -> ("Boolean"=w346:bool)  [unwired: 9 in, 1 out]
        n103 = call-poly <vilib>:"NT Read Value.vi"("Name"="Mode_Shift") -> ("Boolean"=→"Mode_Shift":bool)  [unwired: 9 in, 1 out]
        n104 = call-poly <vilib>:"NT Read Value.vi"("Name"="Mode_Butterfly") -> ("Boolean"=→"Mode_Butterfly":bool)  [unwired: 9 in, 1 out]
        n105 = call-poly <vilib>:"NT Read Value.vi"("Name"="Autopilot_State") -> ("Boolean"=w360:bool)  [unwired: 9 in, 1 out]
        n106 = call-poly <vilib>:"NT Read Value.vi"("Name"="Range_To_Target") -> ("Numeric"=w353:dbl)  [unwired: 9 in, 1 out]
        n107 = call-poly <vilib>:"NT Read Value.vi"("Name"="Compressor_On") -> ("Boolean"=→"Compressor_On":bool)  [unwired: 9 in, 1 out]
        n108 = call "BlinkLight.vi"() -> ("Blinked"=w355:bool)  [unwired: 1 in]
        n109 = call-poly <vilib>:"NT Read Value.vi"("Name"="Range_Color_Left") -> ("Numeric"=w511:dbl)  [unwired: 9 in, 1 out]
        n110 = call-poly <vilib>:"NT Read Value.vi"("Name"="Range_Color_Back") -> ("Numeric"=w517:dbl)  [unwired: 9 in, 1 out]
        n111 = call-poly <vilib>:"NT Read Value.vi"("Name"="Range_Color_Front-Right") -> ("Numeric"=w515:dbl)  [unwired: 9 in, 1 out]
        n112 = call-poly <vilib>:"NT Read Value.vi"("Name"="Range_Color_Right") -> ("Numeric"=w513:dbl)  [unwired: 9 in, 1 out]
        n113 = call-poly <vilib>:"NT Read Value.vi"("Name"="Range_Color_Front-Left") -> ("Numeric"=w465:dbl)  [unwired: 9 in, 1 out]
        n114 = Select(t=TRUE, s=w346, f=w355) -> (s? t:f=w358:bool)
        n115 = Select(t=w353, s=w346, f=0.0) -> (s? t:f=w351:dbl)
        n116 = Select(t=w358, s=w360, f=FALSE) -> (s? t:f=→"Autopilot":bool)
        n117 = To Unsigned Long Integer(number=w511) -> (unsigned 32bit integer=→"Range_Color_Left":u32)
        n118 = To Unsigned Long Integer(number=w517) -> (unsigned 32bit integer=→"Range_Color_Back":u32)
        n119 = To Unsigned Long Integer(number=w515) -> (unsigned 32bit integer=→"Range_Color_Front-Right":u32)
        n120 = To Unsigned Long Integer(number=w513) -> (unsigned 32bit integer=→"Range_Color_Right":u32)
        n121 = To Unsigned Long Integer(number=w465) -> (unsigned 32bit integer=→"Range_Color_Front-Left":u32)
        n122 = Round To Nearest(number=w351) -> (nearest integer value=w350:dbl)
        n123 = To Word Integer(number=w350) -> (16bit integer=w349:i16)
        n124 = call-poly <vilib>:"NT Read Value.vi"("Name"="Hatch_Ejection_State") -> ("Boolean"=→"Hatch_Ejection_State":bool)  [unwired: 9 in, 1 out]
        n125 = Negate(x=w349) -> (-x=w347:i16)
        n126 = call-poly <vilib>:"NT Read Value.vi"("Name"="Capture_Cargo") -> ("Boolean"=→"Capture_Cargo":bool)  [unwired: 9 in, 1 out]
        n127 = call-poly <vilib>:"NT Read Value.vi"("Name"="Capture_Hatch") -> ("Boolean"=→"Capture_Hatch":bool)  [unwired: 9 in, 1 out]
        n128 = Select(t=w347, s=w346, f=i16 -200) -> (s? t:f=→"Range_to_Target (L)" →"Range_to_Target (R)":i16)
        n129 = call-poly <vilib>:"NT Read Value.vi"("Name"="COM_Warning") -> ("Boolean"=→"COM_Warning":bool)  [unwired: 9 in, 1 out]
        n130 = call-poly <vilib>:"NT Read Value.vi"("Name"="Tilt_Interlock") -> ("Boolean"=→"Tilt_Interlock":bool)  [unwired: 9 in, 1 out]
        n131 = call-poly <vilib>:"NT Read Value.vi"("Name"="Climb_Sequence") -> ("String"=→"Climb_Sequence":string)  [unwired: 9 in, 1 out]
        n132 = call-poly <vilib>:"NT Read Value.vi"("Name"="Hatch_Rocket_2_Light") -> ("Boolean"=w269:bool)  [unwired: 9 in, 1 out]
        n133 = call-poly <vilib>:"NT Read Value.vi"("Name"="Hatch_Feeder_Light") -> ("Boolean"=w267:bool)  [unwired: 9 in, 1 out]
        n134 = call-poly <vilib>:"NT Read Value.vi"("Name"="Hatch_Ground_Light") -> ()  [unwired: 9 in, 2 out]
        n135 = call-poly <vilib>:"NT Read Value.vi"("Name"="Hatch_Rocket_3_Light") -> ("Boolean"=w271:bool)  [unwired: 9 in, 1 out]
        n136 = call-poly <vilib>:"NT Read Value.vi"("Name"="Hatch_Rocket_1_Light") -> ("Boolean"=w270:bool)  [unwired: 9 in, 1 out]
        n137 = call-poly <vilib>:"NT Read Value.vi"("Name"="Hatch_Ship_Light") -> ("Boolean"=w268:bool)  [unwired: 9 in, 1 out]
        n138 = call-poly <vilib>:"NT Read Value.vi"("Name"="Cargo_Rocket_3_Light") -> ("Boolean"=w252:bool)  [unwired: 9 in, 1 out]
        n139 = call-poly <vilib>:"NT Read Value.vi"("Name"="Cargo_Rocket_2_Light") -> ("Boolean"=w251:bool)  [unwired: 9 in, 1 out]
        n140 = call-poly <vilib>:"NT Read Value.vi"("Name"="Cargo_Rocket_1_Light") -> ("Boolean"=w250:bool)  [unwired: 9 in, 1 out]
        n141 = call-poly <vilib>:"NT Read Value.vi"("Name"="Cargo_Feeder_Light") -> ("Boolean"=w249:bool)  [unwired: 9 in, 1 out]
        n142 = call-poly <vilib>:"NT Read Value.vi"("Name"="Cargo_Ship_Light") -> ("Boolean"=w215:bool)  [unwired: 9 in, 1 out]
        n143 = call-poly <vilib>:"NT Read Value.vi"("Name"="Elevator_Stow_Light") -> ()  [unwired: 9 in, 2 out]
        n144 = call-poly <vilib>:"NT Read Value.vi"("Name"="Cargo_Ground_Light") -> ("Boolean"=w214:bool)  [unwired: 9 in, 1 out]
        n145 = call-poly <vilib>:"NT Read Value.vi"("Name"="Climb_Light") -> ()  [unwired: 9 in, 2 out]
        n146 = call-poly <vilib>:"NT Read Value.vi"("Name"="Elevator_Encoder_Malfunction") -> ("Boolean"=→"Elevator_Encoder_Malfunction" →"Elevator_Stall":bool)  [unwired: 9 in, 1 out]
        n147 = call-poly <vilib>:"NT Read Value.vi"("Name"="Elevator_Brake_State") -> ("Boolean"=w370:bool)  [unwired: 9 in, 1 out]
        n148 = call-poly <vilib>:"NT Read Value.vi"("Name"="Blink_Elevator_State") -> ("Boolean"=w369:bool)  [unwired: 9 in, 1 out]
        n149 = call-poly <vilib>:"NT Read Value.vi"("Name"="Hatch_Rocket_2_Light") -> ("Boolean"=w424:bool)  [unwired: 9 in, 1 out]
        n150 = call-poly <vilib>:"NT Read Value.vi"("Name"="Hatch_Feeder_Light") -> ("Boolean"=w422:bool)  [unwired: 9 in, 1 out]
        n151 = call-poly <vilib>:"NT Read Value.vi"("Name"="Hatch_Ground_Light") -> ("Boolean"=w421:bool)  [unwired: 9 in, 1 out]
        n152 = call-poly <vilib>:"NT Read Value.vi"("Name"="Hatch_Rocket_3_Light") -> ("Boolean"=w425:bool)  [unwired: 9 in, 1 out]
        n153 = call-poly <vilib>:"NT Read Value.vi"("Name"="Hatch_Rocket_1_Light") -> ("Boolean"=w423:bool)  [unwired: 9 in, 1 out]
        n154 = call-poly <vilib>:"NT Read Value.vi"("Name"="Hatch_Ship_Light") -> ("Boolean"=w420:bool)  [unwired: 9 in, 1 out]
        n155 = call-poly <vilib>:"NT Read Value.vi"("Name"="Cargo_Rocket_3_Light") -> ("Boolean"=w435:bool)  [unwired: 9 in, 1 out]
        n156 = call-poly <vilib>:"NT Read Value.vi"("Name"="Cargo_Rocket_2_Light") -> ("Boolean"=w434:bool)  [unwired: 9 in, 1 out]
        n157 = call-poly <vilib>:"NT Read Value.vi"("Name"="Cargo_Rocket_1_Light") -> ("Boolean"=w433:bool)  [unwired: 9 in, 1 out]
        n158 = call-poly <vilib>:"NT Read Value.vi"("Name"="Cargo_Feeder_Light") -> ("Boolean"=w432:bool)  [unwired: 9 in, 1 out]
        n159 = call-poly <vilib>:"NT Read Value.vi"("Name"="Cargo_Ship_Light") -> ("Boolean"=w438:bool)  [unwired: 9 in, 1 out]
        n160 = call-poly <vilib>:"NT Read Value.vi"("Name"="Elevator_Stow_Light") -> ("Boolean"=w388:bool)  [unwired: 9 in, 1 out]
        n161 = call-poly <vilib>:"NT Read Value.vi"("Name"="Cargo_Ground_Light") -> ("Boolean"=w436:bool)  [unwired: 9 in, 1 out]
        n162 = call-poly <vilib>:"NT Read Value.vi"("Name"="Climb_Light") -> ("Boolean"=w437:bool)  [unwired: 9 in, 1 out]
        n163 = call "BlinkLight.vi"() -> ("Blinked"=w373:bool)  [unwired: 1 in]
        n164 = call "BlinkLight.vi"() -> ("Blinked"=w368:bool)  [unwired: 1 in]
        n165 = Compound Arithmetic op=OR(w252, w251, w250, w249, w214) -> (w247:bool)
        n166 = Compound Arithmetic op=OR(w267, w271, w270, w269, w268, w215) -> (w266:bool)
        n167 = Select(t=w368, s=w369, f=w370) -> (s? t:f=→"Elevator_Brake_State":bool)
        n168 = Select(t=w373, s=w424, f=w374) -> (s? t:f=→"Hatch_Rocket_2_Light":bool)
        n169 = Select(t=w373, s=w422, f=w374) -> (s? t:f=→"Hatch_Feeder_Light":bool)
        n170 = Select(t=w373, s=w421, f=w374) -> (s? t:f=→"Hatch_Ground_Light":bool)
        n171 = Select(t=w373, s=w425, f=w374) -> (s? t:f=→"Hatch_Rocket_3_Light":bool)
        n172 = Select(t=w373, s=w423, f=w374) -> (s? t:f=→"Hatch_Rocket_1_Light":bool)
        n173 = Select(t=w373, s=w420, f=w374) -> (s? t:f=→"Hatch_Ship_Light":bool)
        n174 = Select(t=w373, s=w435, f=w374) -> (s? t:f=→"Cargo_Rocket_3_Light":bool)
        n175 = Select(t=w373, s=w434, f=w374) -> (s? t:f=→"Cargo_Rocket_2_Light":bool)
        n176 = Select(t=w373, s=w433, f=w374) -> (s? t:f=→"Cargo_Rocket_1_Light":bool)
        n177 = Select(t=w373, s=w432, f=w374) -> (s? t:f=→"Cargo_Feeder_Light":bool)
        n178 = Select(t=w373, s=w438, f=w374) -> (s? t:f=→"Cargo_Ship_Light":bool)
        n179 = Select(t=w373, s=w388, f=w374) -> (s? t:f=→"Elevator_Stow_Light":bool)
        n180 = Select(t=w373, s=w436, f=w374) -> (s? t:f=→"Cargo_Ground_Light":bool)
        n181 = Select(t=w373, s=w437, f=w374) -> (s? t:f=→"Climb_Light":bool)
        n182 = local read "LimeLight_Override"() -> (w274:bool)
        n183 = call-poly <vilib>:"NT Read Value.vi"("Name"="At_Climb_Height") -> ("Boolean"=→"At Climb_Height":bool)  [unwired: 9 in, 1 out]
        n184 = call-poly <vilib>:"NT Read Value.vi"("Name"="PTO_Engaged") -> ("Boolean"=→"PTO_Engaged":bool)  [unwired: 9 in, 1 out]
        n185 = call-poly <vilib>:"NT Read Value.vi"("Name"="Elevator_Moving") -> ("Boolean"=w337:bool)  [unwired: 9 in, 1 out]
        n186 = call-poly <vilib>:"NT Read Value.vi"("Name"="Intake_In") -> ("Boolean"=→"Intake_In":bool)  [unwired: 9 in, 1 out]
        n187 = call "BlinkLight.vi"() -> ("Blinked"=w338:bool)  [unwired: 1 in]
        n188 = Not(x=w274) -> (.not. x?=w253:bool)
        n189 = Select(t=w338, s=w337, f=FALSE) -> (s? t:f=→"Elevator_Moving":bool)
        n190 = Compound Arithmetic op=AND(w253, w247) -> (→"Ret_CARGO Left" →"Ret_CARGO Right":bool)
        n191 = Compound Arithmetic op=AND(w253, w266) -> (→"Ret_HATCH Left" →"Ret_HATCH Right":bool)
        n192 = Compound Arithmetic op=AND(w253, FALSE ("value")) -> (→"Ret_CARGO Center":bool)
        n193 = local read "Master_Safety_Override_1"() -> (w316:bool)
        n194 = local read "Master_Safety_Override_2"() -> (w315:bool)
        n195 = local read "Control Loop Time (ms)"() -> (w310:u32)
        n196 = local read "Elevator_Motor_Failure"() -> (w246:bool)
        n197 = call-poly <vilib>:"NT Read Value.vi"("Name"="State_Conflict") -> ("Boolean"=→"State_Conflict":bool)  [unwired: 9 in, 1 out]
        n198 = local read "Check_Limit_Switch"() -> (w220:bool)
        n199 = local read "Super_Test_Mode"() -> (w311:bool)
        n200 = local read "Elevator_Manual"() -> (w312:bool)
        n201 = local read "Elevator_Stall"() -> (w314:bool)
        n202 = local read "Tilt_Interlock"() -> (w313:bool)
        n203 = call-poly <vilib>:"NT Read Value.vi"("Name"="Control_Loop_Time") -> ("Numeric"=w456:dbl)  [unwired: 9 in, 1 out]
        n204 = And(x="Climb", y="Climb_Safety") -> (x .and. y?=w343:bool)
        n205 = call-poly <vilib>:"NT Write Value.vi"("Boolean"="Cargo_Ship", "Name"="Cargo_Ship") -> ()  [unwired: 9 in, 1 out]
        n206 = call-poly <vilib>:"NT Write Value.vi"("Boolean"="Cargo_Feeder", "Name"="Cargo_Feeder") -> ()  [unwired: 9 in, 1 out]
        n207 = call-poly <vilib>:"NT Write Value.vi"("Boolean"="Cargo_Ground", "Name"="Cargo_Ground") -> ()  [unwired: 9 in, 1 out]
        n208 = call-poly <vilib>:"NT Write Value.vi"("Numeric"="Elevator_Kf_2", "Name"="Elevator_Kf_2") -> ()  [unwired: 9 in, 1 out]
        n209 = call-poly <vilib>:"NT Write Value.vi"("Numeric"="Elevator_Kf_1", "Name"="Elevator_Kf_1") -> ()  [unwired: 9 in, 1 out]
        n210 = call-poly <vilib>:"NT Write Value.vi"("Numeric"="Elevator_Kf_3", "Name"="Elevator_Kf_3") -> ()  [unwired: 9 in, 1 out]
        n211 = call-poly <vilib>:"NT Write Value.vi"("Numeric"="Elevator_Kf_Climb", "Name"="Elevator_Kf_Climb") -> ()  [unwired: 9 in, 1 out]
        n212 = call-poly <vilib>:"NT Write Value.vi"("Boolean"="Tilt_Safety_Override", "Name"="Tilt_Safety_Override") -> ()  [unwired: 9 in, 1 out]
        n213 = To Unsigned Long Integer(number=w456) -> (unsigned 32bit integer=→"Control Loop Time (ms)":u32)
        n214 = call-poly <vilib>:"NT Write Value.vi"("Boolean"=w343, "Name"="Climb") -> ()  [unwired: 9 in, 1 out]
        n215 = Greater?(x=w310, y=u32 40) -> (0:w221:bool)
        "Slow_Loop" <- w221
        n216 = And(x=w316, y=w315) -> (x .and. y?=w317:bool)
        n217 = Build Array("N/A") -> (w208:string[])
        n218 = Compound Arithmetic op=OR("Tilt_Safety_Override", w221, w220, w314, w317, w313, w312, w311, w246) -> (w235:bool)
        n219 = call-poly <vilib>:"NT Write Value.vi"("Boolean"="Hatch_Rocket_3", "Name"="Hatch_Rocket_3") -> ()  [unwired: 9 in, 1 out]
        n220 = call-poly <vilib>:"NT Write Value.vi"("Boolean"="Elevator_Stow", "Name"="Elevator_Stow") -> ()  [unwired: 9 in, 1 out]
        n221 = call-poly <vilib>:"NT Read Value.vi"("Default Value"=w208, "Name"="Legal_Drivers") -> ("String Array"=w210:string[])  [unwired: 8 in, 1 out]
        n222 = To Double Precision Float(number="Driver Profile") -> (double precision float=w213:dbl)
        n223 = call-poly <vilib>:"NT Write Value.vi"("Numeric"=w213, "Name"="Selected_Driver") -> ()  [unwired: 9 in, 1 out]
        n224 = property on="Driver Profile" class="Ring (strict)"("Strings []"=w210) -> ()  [unwired: 2 in, 2 out]
        n225 = call-poly <vilib>:"NT Read Value.vi"("Default Value"=0.0, "Name"="Remaining_Time") -> ("Numeric"=w289:dbl)  [unwired: 8 in, 1 out]
        n226 = call "BlinkLight.vi"() -> ("Blinked"=w320:bool)  [unwired: 1 in]
        n227 = Select(t=w320, s=w235, f=FALSE) -> (s? t:f=→"Master_Caution":bool)
        n228 = call-poly <vilib>:"NT Read Value.vi"("Name"="Robot_On_Ground") -> ("Boolean"=→"Robot_On_Ground":bool)  [unwired: 9 in, 1 out]
        n229 = call-poly <vilib>:"NT Read Value.vi"("Name"="Elevator_Motor_Failure") -> ("Boolean"=w222:bool)  [unwired: 9 in, 1 out]
        "Elevator_Motor_Failure" <- w222
        n230 = In Range and Coerce(upper limit=inf, x=w289, lower limit=0.0) -> (coerced(x)=w292:dbl)  [unwired: 1 out]
        n231 = call-poly <vilib>:"NT Write Value.vi"("Boolean"="Hatch_Rocket_2", "Name"="Hatch_Rocket_2") -> ()  [unwired: 9 in, 1 out]
        n232 = call-poly <vilib>:"NT Write Value.vi"("Boolean"="Hatch_Rocket_1", "Name"="Hatch_Rocket_1") -> ()  [unwired: 9 in, 1 out]
        n233 = call-poly <vilib>:"NT Write Value.vi"("Boolean"="Hatch_Ground", "Name"="Hatch_Ground") -> ()  [unwired: 9 in, 1 out]
        n234 = call-poly <vilib>:"NT Write Value.vi"("Boolean"="Hatch_Feeder", "Name"="Hatch_Feeder") -> ()  [unwired: 9 in, 1 out]
        n235 = call-poly <vilib>:"NT Read Value.vi"("Name"="Elevator_1_Current") -> ("Numeric"=w232:dbl)  [unwired: 9 in, 1 out]
        "Elevator_1_Current" <- w232
        n236 = call-poly <vilib>:"NT Read Value.vi"("Name"="Elevator_2_Current") -> ("Numeric"=w231:dbl)  [unwired: 9 in, 1 out]
        "Elevator_2_Current" <- w231
        n237 = call-poly <vilib>:"NT Read Value.vi"("Name"="Elevator_3_Current") -> ("Numeric"=w230:dbl)  [unwired: 9 in, 1 out]
        "Elevator_3_Current" <- w230
        n238 = Build Array("N/A") -> (w193:string[])
        n239 = call-poly <vilib>:"NT Read Value.vi"("Name"="Presure_Leak") -> ("Boolean"=w199:bool)  [unwired: 9 in, 1 out]
        n240 = call-poly <vilib>:"NT Read Value.vi"("Name"="Catastrophic_Pressure_Leak") -> ("Boolean"=w198:bool)  [unwired: 9 in, 1 out]
        n241 = To Single Precision Float(number=w292) -> (single precision float=→"Match Time(s)":sgl)
        n242 = Less?(x=w289, y="Warning Time (s)") -> (x < y?=w295:bool)
        n243 = Greater Than 0?(x=w289) -> (x > 0?=w294:bool)
        n244 = call-poly <vilib>:"NT Read Value.vi"("Name"="Check_Limit_Switch") -> ("Boolean"=→"Check_Limit_Switch":bool)  [unwired: 9 in, 1 out]
        n245 = call-poly <vilib>:"NT Read Value.vi"("Default Value"=w193, "Name"="Legal_Auto_Plays") -> ("String Array"=w191:string[])  [unwired: 8 in, 1 out]
        n246 = And(x=w295, y=w294) -> (x .and. y?=w293:bool)
        n247 = To Double Precision Float(number="Autonomous Play") -> (double precision float=w197:dbl)
        n248 = call-poly <vilib>:"NT Write Value.vi"("Boolean"="Refresh_Auto_Play_List", "Name"="Refresh_Auto_Play_List") -> ()  [unwired: 9 in, 1 out]
        n249 = call "BlinkLight.vi"() -> ("Blinked"=w297:bool)  [unwired: 1 in]
        n250 = call-poly <vilib>:"NT Write Value.vi"("Numeric"=w197, "Name"="Selected_Auto_Play") -> ()  [unwired: 9 in, 1 out]
        n251 = property on="Autonomous Play" class="Ring (strict)"("Strings []"=w191) -> ()  [unwired: 2 in, 2 out]
        n252 = Or(x=w199, y=w198) -> (x .or. y?=→"Pressure_Leak":bool)
        n253 = call "BlinkLight.vi"() -> ("Blinked"=w257:bool)  [unwired: 1 in]
        n254 = Select(t=w297, s=w293, f=FALSE) -> (s? t:f=→"Out_Of_Time":bool)
        n255 = Select(t=w257, s=w222, f=FALSE) -> (s? t:f=→"Elevator_Motor_Failure_2":bool)
        n256 = call-poly <vilib>:"NT Write Value.vi"("Boolean"="Cargo_Rocket_2", "Name"="Cargo_Rocket_2") -> ()  [unwired: 9 in, 1 out]
        n257 = call-poly <vilib>:"NT Write Value.vi"("Boolean"="Cargo_Rocket_1", "Name"="Cargo_Rocket_1") -> ()  [unwired: 9 in, 1 out]
        n258 = Less?(x=w231, y=w229) -> (x < y?=w227:bool)
        n259 = call-poly <vilib>:"NT Write Value.vi"("Boolean"="Cargo_Rocket_3", "Name"="Cargo_Rocket_3") -> ()  [unwired: 9 in, 1 out]
        n260 = Less?(x=w232, y=w229) -> (x < y?=w228:bool)
        n261 = call-poly <vilib>:"NT Write Value.vi"("Boolean"="Hatch_Ship", "Name"="Hatch_Ship") -> ()  [unwired: 9 in, 1 out]
        n262 = Less?(x=w230, y=w229) -> (x < y?=w226:bool)
        n263 = call-poly <vilib>:"NT Read Value.vi"("Name"="Robot_Off_Ground") -> ("Boolean"=→"Robot_Off_Ground":bool)  [unwired: 9 in, 1 out]
        n264 = Compound Arithmetic op=AND(w227, w222) -> (→"E2 Warning":bool)
        n265 = Compound Arithmetic op=AND(w226, w222) -> (→"E3 Warning":bool)
        n266 = Compound Arithmetic op=AND(w228, w222) -> (→"E1 Warning":bool)
        n267 = call-poly <vilib>:"NT Read Value.vi"("Name"="Range_Front-Left") -> ("Numeric"=→"Range_Front-Left":dbl)  [unwired: 9 in, 1 out]
        n268 = call-poly <vilib>:"NT Read Value.vi"("Name"="Range_Back") -> ("Numeric"=→"Range_Back":dbl)  [unwired: 9 in, 1 out]
        n269 = call-poly <vilib>:"NT Read Value.vi"("Name"="Right_Drive_Vel") -> ("Numeric"=→"Right_Drive_Vel":dbl)  [unwired: 9 in, 1 out]
        n270 = call-poly <vilib>:"NT Read Value.vi"("Name"="Elevator_Goal") -> ("Numeric"=→"Elevator_Goal_Visual":dbl)  [unwired: 9 in, 1 out]
        n271 = call-poly <vilib>:"NT Read Value.vi"("Name"="Range_Left") -> ("Numeric"=→"Range_Left":dbl)  [unwired: 9 in, 1 out]
        n272 = call-poly <vilib>:"NT Read Value.vi"("Name"="Elevator_Pos") -> ("Numeric"=→"Elevator_Pos" →"Elevator_Pos_Visual":dbl)  [unwired: 9 in, 1 out]
        n273 = call-poly <vilib>:"NT Read Value.vi"("Name"="Battery_Voltage") -> ("Numeric"=w239:dbl)  [unwired: 9 in, 1 out]
        "Battery_Voltage" <- w239
        n274 = call-poly <vilib>:"NT Write Value.vi"("Boolean"="Vision_Target_L_R", "Name"="Vision_Target_L_R") -> ()  [unwired: 9 in, 1 out]
        n275 = call-poly <vilib>:"NT Write Value.vi"("Numeric"="Vacuum_Pump", "Name"="Vacuum_Pump") -> ()  [unwired: 9 in, 1 out]
        n276 = call-poly <vilib>:"NT Write Value.vi"("Boolean"="Reinit_Stow_Vacuum", "Name"="Reinit_Stow_Vacuum") -> ()  [unwired: 9 in, 1 out]
        n277 = call "TimeBelowThreshold.vi"("Current Value"=w239, "Threshold"=11.0 ("y")) -> ("Time Below"=w237:u32)  [unwired: 3 in]
        n278 = call-poly <vilib>:"NT Write Value.vi"("Boolean"="Super_Test_Mode", "Name"="Super_Test_Mode") -> ()  [unwired: 9 in, 1 out]
        n279 = call-poly <vilib>:"NT Write Value.vi"("Boolean"="Master_Safety_Override_2", "Name"="Master_Safety_Override_2") -> ()  [unwired: 9 in, 1 out]
        n280 = call-poly <vilib>:"NT Write Value.vi"("Boolean"="Master_Safety_Override_1", "Name"="Master_Safety_Override_1") -> ()  [unwired: 9 in, 1 out]
        n281 = call-poly <vilib>:"NT Write Value.vi"("Boolean"="Elevator_Manual", "Name"="Elevator_Manual") -> ()  [unwired: 9 in, 1 out]
        n282 = Greater?(x=w237, y=u32 2000) -> (0:→"Battery_Critical":bool)
        n283 = local read "Dashboard Tab"() -> (w367:T1)
        n284 = call-poly <vilib>:"NT Read Value.vi"("Name"="Range_Right") -> ("Numeric"=→"Range_Right":dbl)  [unwired: 9 in, 1 out]
        n285 = call-poly <vilib>:"NT Read Value.vi"("Name"="Tank_Pressure") -> ("Numeric"=→"Tank_Pressure" →"Pressure_Visualize":dbl)  [unwired: 9 in, 1 out]
        n286 = call-poly <vilib>:"NT Read Value.vi"("Name"="Left_Drive_Vel") -> ("Numeric"=→"Left_Drive_Vel":dbl)  [unwired: 9 in, 1 out]
        n287 = call-poly <vilib>:"NT Read Value.vi"("Name"="Range_Front-Right") -> ("Numeric"=→"Range_Front-Right":dbl)  [unwired: 9 in, 1 out]
        n288 = call-poly <vilib>:"NT Read Value.vi"("Name"="Left_Drive_Pos") -> ("Numeric"=→"Left_Drive_Pos":dbl)  [unwired: 9 in, 1 out]
        n289 = call-poly <vilib>:"NT Read Value.vi"("Name"="Right_Drive_Pos") -> ("Numeric"=→"Right_Drive_Pos":dbl)  [unwired: 9 in, 1 out]
        n290 = call-poly <vilib>:"NT Read Value.vi"("Name"="Elevator_Power") -> ("Numeric"=→"Elevator_Power":dbl)  [unwired: 9 in, 1 out]
        n291 = To Double Precision Float(number="Climb_Level") -> (double precision float=w244:dbl)
        n292 = call-poly <vilib>:"NT Write Value.vi"("Boolean"="Overclock", "Name"="Overclock") -> ()  [unwired: 9 in, 1 out]
        n293 = call-poly <vilib>:"NT Read Value.vi"("Name"="Ground_Height") -> ("Numeric"=→"Ground_Height":dbl)  [unwired: 9 in, 1 out]
        n294 = Equal?(x=w367, y=T13."Tune") -> (x = y?=w365:bool)
        n295 = call-poly <vilib>:"NT Write Value.vi"("Boolean"="Defense_Driving", "Name"="Defense_Driving") -> ()  [unwired: 9 in, 1 out]
        n296 = call-poly <vilib>:"NT Write Value.vi"("Boolean"="LimeLight_Override", "Name"="LimeLight_Override") -> ()  [unwired: 9 in, 1 out]
        n297 = call-poly <vilib>:"NT Write Value.vi"("Numeric"=w244, "Name"="Climb_Level") -> ()  [unwired: 9 in, 1 out]
        n298 = call-poly <vilib>:"NT Write Value.vi"("Boolean"="Drive_Encoder_Reset", "Name"="Drive_Encoder_Reset") -> ()  [unwired: 9 in, 1 out]
        n299 = call-poly <vilib>:"NT Write Value.vi"("Boolean"=w365, "Name"="Tune_Tab") -> ()  [unwired: 9 in, 1 out]
      }
    }
  }
  n300 = control-ref of="Test Tree"() -> (w34:refnum<vi>)
  n301 = call "Initialize Camera and CheckList.vi"("ListBox in"=w20) -> ()  [unwired: 11 in]
  n302 = Index Array(array=w33) -> (element=w31:refnum<vi>)  [unwired: 1 in]
  n303 = vi-ref "Playback Controls.vi"() -> (w30:refnum<vi>)
  n304 = while {
    tunnel: w31 -> [w520]
    i -> [w523]
    stop <- FALSE stop-if-true
    n305 = Wait (ms)(milliseconds to wait=u32 100) -> ()  [unwired: 1 out]
    n306 = case shown="\"Playback\"" "Rec Mode" {
      tunnel: w523 -> [_ _ w538]
      tunnel: [u32 2829099 ("Base Color") u32 11141120 ("Target Color") w527] -> w519
      frame "Stop", Default {
        # "Reset the color, extra updates don't cost much"
      }
      frame "Record" {
      }
      frame "Playback" {
        # "Playback"
        n307 = Quotient & Remainder(x=w538, y=u32 50 ("milliseconds to wait")) -> (x-y*floor(x/y)=w534:u32)  [unwired: 1 out]
        n308 = Divide(x=w534, y=u32 50 ("milliseconds to wait")) -> (x/y=w531:dbl)
        n309 = Multiply(x=6.283185307179586, y=w531) -> (x*y=w536:dbl)
        n310 = Sine(x=w536) -> (sin(x)=w535:dbl)
        n311 = Absolute Value(x=w535) -> (abs(x)=w528:dbl)
        n312 = call "Interpolate RGB Color.vi"("Proportion"=w528, "Target Color"=u32 30976, "Base Color"=u32 2829099) -> ("Result Color"=w527:u32)  [unwired: 8 in]
      }
    }
    n313 = property class="Pane"(reference=w520, "PaneColor"=w519) -> ()  [unwired: 1 in, 2 out]
  }
  n314 = while {
    tunnel: [w548] -> _
    tunnel: w34 -> [w547]
    tunnel: w30 -> [w546]
    tunnel: w29 -> [w545]
    tunnel: w28 -> [_]
    tunnel: w24 -> [w544]
    tunnel: w12 -> [w543]
    tunnel: w11 -> [w542]
    shift-right: [w541] -> _
    shift-left: _ -> [w540]
    tunnel: w9 -> [w539]
    i -> [w548]
    stop <- FALSE stop-if-true
    n315 = event shown="[0] Timeout" {
      selector: w545 -> [_ _ _ _ _ _ _ _ _ _ _ _ _ _ _ _ _ _ _ _ _]
      dyn-events: [_ _ _ _ _ _ _ _ _ _ _ _ _ _ _ _ w806 _ _ _ _] -> _
      timeout: u32 60 ("milliseconds to wait") -> [_ _ _ _ _ _ _ _ _ _ _ _ _ _ _ _ _ _ _ _ _]
      tunnel: w547 -> [w560 _ _ _ _ _ _ _ _ _ _ _ _ _ _ _ _ _ _ _ _]
      tunnel: "Test Tree" -> [_ _ _ _ _ _ _ _ _ _ _ w775 w783 w785 w789 w797 _ _ _ _ _]
      tunnel: w546 -> [_ _ _ _ _ _ _ _ _ _ _ _ _ _ _ _ w808 _ w826 _ _]
      tunnel: w544 -> [_ _ _ _ _ _ _ _ _ _ _ _ _ _ _ _ w804 _ _ _ _]
      tunnel: w543 -> [_ _ _ _ _ _ _ _ _ _ _ _ _ _ _ _ w802 _ _ _ _]
      tunnel: w542 -> [w555 _ _ _ _ _ w726 _ _ _ _ _ _ _ _ _ _ _ _ _ _]
      tunnel: [w554 w603 w705 w710 w719 w723 w724 w733 w743 w750 w762 w774 w781 w784 w788 w796 w801 w821 w823 w827 w840] -> w541
      tunnel: w540 -> [w554 w603 w705 w710 w719 w723 w724 _ _ w750 w762 w774 w781 w784 w788 w796 w801 w821 w823 w827 w840]
      tunnel: w539 -> [w552 _ _ _ _ _ _ _ _ _ _ _ _ _ _ _ _ _ _ _ _]
      event Timeout {
        n316 = event-data() -> ()  [unwired: 1 in, 1 out]
        n317 = local read "Mode"() -> (w557:T5)
        n318 = case shown="\"Commands\"" "Dashboard Tab" {
          tunnel: w560 -> [_ _ w576 _ _]
          tunnel: "TestMode/Automatic/" ("Name Pattern") -> [_ _ w575 _ _]
          tunnel: T18 [{"Operation"=enum."Clear", "Color Box"=14013909}, {"Operation"=enum."Clear", "Color Box"=14013909}, {"Operation"=enum."Clear", "Color Box"=14013909}, {"Operation"=enum."Clear", "Color Box"=14013909}, {"Operation"=enum."Update", "Color Box"=14013909}, {"Operation"=enum."Update", "Color Box"=16777215}, {"Operation"=enum."Clear", "Color Box"=14013909}, {"Operation"=enum."Clear", "Color Box"=14013909}, {"Operation"=enum."Clear", "Color Box"=14013909}] -> [_ _ w568 _ w596]
          tunnel: w557 -> [_ _ w567 _ w595]
          tunnel: u32[] [15790320, 15790320, 15790320, 15790320, 16777215, 16777215, 15790320, 15790320, 15790320] -> [_ _ _ _ w601]
          tunnel: w555 -> [_ _ _ _ w589]
          tunnel: w552 -> [_ w562 _ _ _]
          frame "TeleOp", Default {
          }
          frame "Tune" {
            n319 = call <vilib>:"WPI_DashboardUpdateNames.vi"("Controls on Tab"=w562) -> ()  [unwired: 11 in]
          }
          frame "Test" {
            w574 = -2 ("Active Item:Row Number")
            n320 = Index Array(array=w568, index=w567) -> (element=w569:T21)
            n321 = Unbundle(w569) -> ("Operation"=w570:enum16{"Update", "Clear"}, "Color Box"=w571:u32)
            n322 = call <vilib>:"NT Read String.vi"("Name"="TestMode/TestName") -> ("String"=w565:string)  [unwired: 9 in, 1 out]
            n323 = call <vilib>:"NT Read and Format Entries as Tree.vi"("Operation"=w570, "Name Pattern"=w575, "Tree Refnum"=w576) -> ()  [unwired: 7 in, 2 out]
            n324 = case shown="\"\"" w565 {
              tunnel: "TestMode/TestProgress" ("Name") -> [w578 _]
              tunnel: "TestMode/TestProgressText" ("Name") -> [w577 _]
              frame Default {
                n325 = call <vilib>:"NT Read Number.vi"("Name"=w578) -> ("Numeric"=w579:dbl)  [unwired: 9 in, 1 out]
                n326 = call <vilib>:"NT Read String.vi"("Name"=w577) -> ("String"=w580:string)  [unwired: 9 in, 1 out]
                n327 = Bundle("Numeric"=w579, "String"=w580) -> (→"Progress":cluster{"Numeric":dbl, "String":string})  [unwired: 1 in]
              }
              frame "" {
                n328 = property on="Progress" class="Clust (strict)"("Visible"=FALSE) -> ()  [unwired: 2 in, 2 out]
                n329 = local write "Test Name"(u16 0) -> ()
              }
            }
            n330 = property on="Test Tree" class="Tree (strict)"("Active Item Row Number"=w574, "ActiveColNum"=w574, "CellBG"=w571, "Active Item Row Number"=-1 ("Active Item:Row Number"), "CellBG"=u32 5789784 ("Color Box")) -> ()  [unwired: 2 in, 2 out]
          }
          frame "Variables" {
            w586 = string[] ["CameraPublisher", "Usage", "DB"]  # Items to initially close
            n331 = First Call?() -> (First Call?: T/F=w587:bool)
            n332 = control-ref of="Tree"() -> (w588:refnum<vi>)
            n333 = Select(t=w586, s=w587, f=string[] []) -> (s? t:f=w584:string[])
            n334 = call <vilib>:"NT Read and Format Entries as Tree.vi"("Tags to  Close"=w584, "Tree Refnum"=w588) -> ()  [unwired: 8 in, 2 out]
          }
          frame "Commands" {
            w597 = u32 5789784 ("Color Box")
            w598 = T22 {"Row"=-1, "Column"=-2} ("Active Cell:Active Cell")
            w600 = T22 {"Row"=-2, "Column"=-2} ("Active Cell:Active Cell")
            n335 = Index Array(array=w601, index=w595) -> (element=w599:u32)
            n336 = Index Array(array=w596, index=w595) -> (element=w594:T21)
            n337 = Unbundle(w594) -> ("Operation"=w593:enum16{"Update", "Clear"})  [unwired: 1 out]
            n338 = local read "Command Selection"() -> (w592:i32)
            n339 = property on="Command Selection" class="MCListbox (strict)"("ActiveCell"=w600, "CellBG"=w599, "ActiveCell"=w598, "CellBG"=w597) -> ()  [unwired: 2 in, 2 out]
            n340 = call <vilib>:"WPI_DashboardUpdate RPC Info.vi"("Operation"=w593) -> ("update"=w591:bool, "commands"=w590:string[][])  [unwired: 9 in]
            n341 = property on="Command Selection" class="MCListbox (strict)"("ItemNames"=w590) -> ()  [unwired: 2 in, 2 out]
            n342 = property on="Command Params" class="Tbl (strict)"("Active Cell"=w600, "Cell BG Color"=w599, "Active Cell"=w598, "Cell BG Color"=w597) -> ()  [unwired: 2 in, 2 out]
            n343 = call <vilib>:"WPI_DashboardUpdate Command Params.vi"("Update"=w591, "NewVal"=w592, "Commands"=w590, "Param Tbl"=w589) -> ()  [unwired: 7 in, 1 out]
          }
        }
        n344 = call <vilib>:"Connextion Info.vi"() -> ("Connected"=→"NT Connection":bool)  [unwired: 10 in, 1 out]
      }
      event "Test Tree": Value Change {
        # "Show appropriate\ncontrols"
        n345 = event-data() -> ("CtlRef"=w606:refnum<vi>, "NewVal"=w604:string)  [unwired: 1 in]
        n346 = call <vilib>:"WPI_UtilitiesGetTreeIOName.vi"("NewVal"=w604, "TreeControl in"=w606) -> ("I/O Name"=w607:string)  [unwired: 9 in]
        n347 = case shown="\"Analog Out\", \"Motor\", \"PWM\"" w607 {
          selector: w607 -> [_ w614 _ w636 w645 _]
          tunnel: w604 -> [_ _ w633 w635 _ w652]
          tunnel: cluster{string[]}[] [{["640x480", "320x240", "160x120"]}, {["Auto", "Fixed indoor", "Fixed outdoor 1", "Fixed outdoor 2", "Fixed fluorescent 1", "Fixed fluorescent 2", "Hold current"]}, {["Auto", "Flicker-free 50 Hz", "Flicker-free 60 Hz", "Hold current"]}, {["None", "Prioritize frame rate", "Prioritize image quality"]}, {["Monochrome", "Color"]}] -> [_ _ _ _ _ w651]
          frame Default {
            w609 = FALSE ("Visible")
            w608 = FALSE ("Visible")
            n348 = property on="Motor" class="Clust (strict)"("Visible"=w608) -> ()  [unwired: 2 in, 2 out]
            n349 = property on="Test Ring" class="Ring (strict)"("Visible"=w608) -> ()  [unwired: 2 in, 2 out]
            n350 = property on="Rev/Fwd" class="Clust (strict)"("Visible"=w609) -> ()  [unwired: 2 in, 2 out]
            n351 = property on="On/Off" class="Bool (strict)"("Visible"=w609) -> ()  [unwired: 2 in, 2 out]
            n352 = property on="Test Slider" class="Slide (strict)"("Visible"=w609) -> ()  [unwired: 2 in, 2 out]
          }
          frame "Analog Out", "Motor", "PWM" {
            w615 = FALSE ("Visible")
            n353 = case shown="\"Analog Out\"" w614 {
              tunnel: [1.0 ("Value") -1.0 ("Value") 0.0 ("Value")] -> w613
              tunnel: [255.0 ("Value") 1.0 ("Value") 5.0 ("Value")] -> w612
              tunnel: [128.0 ("Value") 0.0 ("Value") 0.0 ("Value")] -> w611
              tunnel: [64.0 ("Value") 0.5 ("Value") 1.0 ("Value")] -> w610
              frame "PWM" {
              }
              frame "Motor", Default {
              }
              frame "Analog Out" {
              }
            }
            n354 = property on="Motor" class="Clust (strict)"("Visible"=TRUE) -> ()  [unwired: 2 in, 2 out]
            n355 = property on="Value" class="Slide (strict)"("Value"=w611, "Scale.Minimum"=w613, "Scale.Maximum"=w612, "Scale.Increment"=w610) -> ()  [unwired: 2 in, 2 out]
            n356 = property on="On/Off" class="Bool (strict)"("Visible"=w615) -> ()  [unwired: 2 in, 2 out]
            n357 = property on="Test Slider" class="Slide (strict)"("Visible"=w615) -> ()  [unwired: 2 in, 2 out]
            n358 = property on="Test Ring" class="Ring (strict)"("Visible"=w615) -> ()  [unwired: 2 in, 2 out]
            n359 = property on="Rev/Fwd" class="Clust (strict)"("Visible"=w615) -> ()  [unwired: 2 in, 2 out]
          }
          frame "Servo" {
            w631 = FALSE ("Visible")
            n360 = call <vilib>:"NT Read Number.vi"("Name"=w633) -> ("Numeric"=w632:dbl)  [unwired: 9 in, 1 out]
            n361 = property on="Test Slider" class="Slide (strict)"("Visible"=TRUE, "Scale.Maximum"=170.0 ("Scale.Range:Maximum")) -> ()  [unwired: 2 in, 2 out]
            n362 = local write "Test Slider"(w632) -> ()
            n363 = property on="Motor" class="Clust (strict)"("Visible"=w631) -> ()  [unwired: 2 in, 2 out]
            n364 = property on="Rev/Fwd" class="Clust (strict)"("Visible"=w631) -> ()  [unwired: 2 in, 2 out]
            n365 = property on="On/Off" class="Bool (strict)"("Visible"=w631) -> ()  [unwired: 2 in, 2 out]
            n366 = property on="Test Ring" class="Ring (strict)"("Visible"=w631) -> ()  [unwired: 2 in, 2 out]
          }
          frame "Relay", "Solenoid" {
            w634 = FALSE ("Visible")
            n367 = property on="Motor" class="Clust (strict)"("Visible"=w634) -> ()  [unwired: 2 in, 2 out]
            n368 = property on="Test Slider" class="Slide (strict)"("Visible"=w634) -> ()  [unwired: 2 in, 2 out]
            n369 = Search and Replace String(input string=w635, search string="/Value  **", replace string="/Direction") -> (result string=w641:string)  [unwired: 5 in, 3 out]
            n370 = property on="Test Ring" class="Ring (strict)"("Visible"=w634) -> ()  [unwired: 2 in, 2 out]
            n371 = call <vilib>:"NT Read String.vi"("Name"=w641) -> ("String"=w639:string)  [unwired: 9 in, 1 out]
            n372 = Equal?(x="Both directions", y=w639) -> (x = y?=w637:bool)
            n373 = Not(x=w637) -> (.not. x?=w638:bool)
            n374 = property on="Rev/Fwd" class="Clust (strict)"("Visible"=w637) -> ()  [unwired: 2 in, 2 out]
            n375 = property on="On/Off" class="Bool (strict)"("Visible"=w638, "Caption.Text"=w636) -> ()  [unwired: 2 in, 2 out]
          }
          frame "Compressor", "Digital Out" {
            w644 = FALSE ("Visible")
            # "Get direction and finish"
            n376 = property on="Motor" class="Clust (strict)"("Visible"=w644) -> ()  [unwired: 2 in, 2 out]
            n377 = property on="Test Slider" class="Slide (strict)"("Visible"=w644) -> ()  [unwired: 2 in, 2 out]
            n378 = property on="Test Ring" class="Ring (strict)"("Visible"=w644) -> ()  [unwired: 2 in, 2 out]
            n379 = property on="On/Off" class="Bool (strict)"("Visible"=TRUE, "Caption.Text"=w645) -> ()  [unwired: 2 in, 2 out]
            n380 = property on="Rev/Fwd" class="Clust (strict)"("Visible"=FALSE) -> ()  [unwired: 2 in, 2 out]
          }
          frame "Camera" {
            n381 = call <vilib>:"Get Last Path Segment.vi"("String in"=w652) -> ("String out"=w653:string)  [unwired: 10 in]
            n382 = property on="On/Off" class="Bool (strict)"("Visible"=FALSE) -> ()  [unwired: 2 in, 2 out]
            n383 = property on="Motor" class="Clust (strict)"("Visible"=FALSE) -> ()  [unwired: 2 in, 2 out]
            n384 = property on="Rev/Fwd" class="Clust (strict)"("Visible"=FALSE) -> ()  [unwired: 2 in, 2 out]
            n385 = case shown="\"White Balance  **\"" w653 {
              tunnel: w652 -> [w659 w668 w677 w686 w695 _ w701]
              tunnel: w651 -> [w657 w665 w674 w683 w692 _ _]
              frame "Size  **" {
                n386 = Index Array(array=w657) -> (element=w656:cluster{string[]})  [unwired: 1 in]
                n387 = call <vilib>:"NT Read String.vi"("Name"=w659) -> ("String"=w658:string)  [unwired: 9 in, 1 out]
                n388 = Unbundle(w656) -> (w654:string[])
                n389 = Match First String(2:w654, 3:w658) -> (0:w655:i32)  [unwired: 1 out]
                n390 = property on="Test Ring" class="Ring (strict)"("Value"=w655, "Strings []"=w654) -> ()  [unwired: 2 in, 2 out]
                n391 = property on="Test Ring" class="Ring (strict)"("Visible"=TRUE) -> ()  [unwired: 2 in, 2 out]
                n392 = property on="Test Slider" class="Slide (strict)"("Visible"=FALSE) -> ()  [unwired: 2 in, 2 out]
              }
              frame "White Balance  **" {
                n393 = Index Array(array=w665, index=1) -> (element=w666:cluster{string[]})
                n394 = call <vilib>:"NT Read String.vi"("Name"=w668) -> ("String"=w667:string)  [unwired: 9 in, 1 out]
                n395 = Unbundle(w666) -> (w663:string[])
                n396 = Match First String(2:w663, 3:w667) -> (0:w662:i32)  [unwired: 1 out]
                n397 = property on="Test Ring" class="Ring (strict)"("Value"=w662, "Strings []"=w663) -> ()  [unwired: 2 in, 2 out]
                n398 = property on="Test Ring" class="Ring (strict)"("Visible"=TRUE) -> ()  [unwired: 2 in, 2 out]
                n399 = property on="Test Slider" class="Slide (strict)"("Visible"=FALSE) -> ()  [unwired: 2 in, 2 out]
              }
              frame "Exposure  **" {
                n400 = Index Array(array=w674, index=2) -> (element=w675:cluster{string[]})
                n401 = call <vilib>:"NT Read String.vi"("Name"=w677) -> ("String"=w676:string)  [unwired: 9 in, 1 out]
                n402 = Unbundle(w675) -> (w671:string[])
                n403 = Match First String(2:w671, 3:w676) -> (0:w672:i32)  [unwired: 1 out]
                n404 = property on="Test Ring" class="Ring (strict)"("Value"=w672, "Strings []"=w671) -> ()  [unwired: 2 in, 2 out]
                n405 = property on="Test Ring" class="Ring (strict)"("Visible"=TRUE) -> ()  [unwired: 2 in, 2 out]
                n406 = property on="Test Slider" class="Slide (strict)"("Visible"=FALSE) -> ()  [unwired: 2 in, 2 out]
              }
              frame "Exposure Priority  **" {
                n407 = Index Array(array=w683, index=3) -> (element=w684:cluster{string[]})
                n408 = call <vilib>:"NT Read String.vi"("Name"=w686) -> ("String"=w685:string)  [unwired: 9 in, 1 out]
                n409 = Unbundle(w684) -> (w680:string[])
                n410 = Match First String(2:w680, 3:w685) -> (0:w681:i32)  [unwired: 1 out]
                n411 = property on="Test Ring" class="Ring (strict)"("Value"=w681, "Strings []"=w680) -> ()  [unwired: 2 in, 2 out]
                n412 = property on="Test Ring" class="Ring (strict)"("Visible"=TRUE) -> ()  [unwired: 2 in, 2 out]
                n413 = property on="Test Slider" class="Slide (strict)"("Visible"=FALSE) -> ()  [unwired: 2 in, 2 out]
              }
              frame "Color Enable  **" {
                n414 = Index Array(array=w692, index=4) -> (element=w693:cluster{string[]})
                n415 = call <vilib>:"NT Read String.vi"("Name"=w695) -> ("String"=w694:string)  [unwired: 9 in, 1 out]
                n416 = Unbundle(w693) -> (w689:string[])
                n417 = Match First String(2:w689, 3:w694) -> (0:w690:i32)  [unwired: 1 out]
                n418 = property on="Test Ring" class="Ring (strict)"("Value"=w690, "Strings []"=w689) -> ()  [unwired: 2 in, 2 out]
                n419 = property on="Test Ring" class="Ring (strict)"("Visible"=TRUE) -> ()  [unwired: 2 in, 2 out]
                n420 = property on="Test Slider" class="Slide (strict)"("Visible"=FALSE) -> ()  [unwired: 2 in, 2 out]
              }
              frame Default {
                n421 = property on="Test Ring" class="Ring (strict)"("Visible"=FALSE) -> ()  [unwired: 2 in, 2 out]
                n422 = property on="Test Slider" class="Slide (strict)"("Visible"=FALSE) -> ()  [unwired: 2 in, 2 out]
              }
              frame "Brightness  **", "Color Level  **", "Compression  **", "FPS  **", "Sharpness  **" {
                n423 = call <vilib>:"NT Read Number.vi"("Name"=w701) -> ("Numeric"=w700:dbl)  [unwired: 9 in, 1 out]
                n424 = local write "Test Slider"(w700) -> ()
                n425 = property on="Test Slider" class="Slide (strict)"("Visible"=TRUE, "Scale.Maximum"=100.0 ("Scale.Range:Maximum")) -> ()  [unwired: 2 in, 2 out]
                n426 = property on="Test Ring" class="Ring (strict)"("Visible"=FALSE) -> ()  [unwired: 2 in, 2 out]
              }
            }
          }
        }
        n427 = property on="Progress" class="Clust (strict)"("Visible"=FALSE) -> ()  [unwired: 2 in, 2 out]
      }
      event "Test Name": Mouse Enter {
        # "Populate the ring with the list of tests"
        n428 = event-data() -> ()  [unwired: 1 in, 1 out]
        n429 = call <vilib>:"NT Read String Array.vi"("Name"="TestMode/TestList") -> ("String Array"=w709:string[])  [unwired: 9 in, 1 out]
        n430 = Build Array (concatenate)("Select the test to run...", w709) -> (w708:string[])
        n431 = property on="Test Name" class="Ring (strict)"("Strings []"=w708) -> ()  [unwired: 2 in, 2 out]
      }
      event "Test Name": Value Change {
        w711 = FALSE ("Visible")
        # "Tell the robot the test name to run"
        n432 = event-data() -> ("NewVal"=w715:u16)  [unwired: 1 in]
        n433 = property on="Test Name" class="Ring (strict)"() -> ("Strings []"=w716:string[])  [unwired: 2 in, 2 out]
        n434 = local write "Progress"(T6 {"Test Progress"=0, "Test Progress Text"=""} ("Progress")) -> ()
        n435 = Index Array(array=w716, index=w715) -> (element=w714:string)
        n436 = call <vilib>:"NT Write String.vi"("String"=w714, "Name"="TestMode/TestName") -> ()  [unwired: 9 in, 1 out]
        n437 = property on="Progress" class="Clust (strict)"("Visible"=TRUE) -> ()  [unwired: 2 in, 2 out]
        n438 = property on="Motor" class="Clust (strict)"("Visible"=w711) -> ()  [unwired: 2 in, 2 out]
        n439 = property on="Test Slider" class="Slide (strict)"("Visible"=w711) -> ()  [unwired: 2 in, 2 out]
        n440 = property on="On/Off" class="Bool (strict)"("Visible"=w711) -> ()  [unwired: 2 in, 2 out]
        n441 = property on="Rev/Fwd" class="Clust (strict)"("Visible"=w711) -> ()  [unwired: 2 in, 2 out]
        n442 = property on="Test Ring" class="Ring (strict)"("Visible"=w711) -> ()  [unwired: 2 in, 2 out]
      }
      event "Select Auto": Mouse Enter {
        # "Populate the combo box with the list of autonomous options"
        n443 = event-data() -> ()  [unwired: 1 in, 1 out]
        n444 = call <vilib>:"NT Read String Array.vi"("Name"="Auto List") -> ("String Array"=w718:string[])  [unwired: 9 in, 1 out]
        n445 = property on="Select Auto" class="CmbBox"("Strings[]"=w718) -> ()  [unwired: 2 in, 2 out]
      }
      event "Select Auto": Value Change {
        # "User modified the Auto Selection. Write to NT variable so robot knows."
        n446 = event-data() -> ("NewVal"=w721:string)  [unwired: 1 in]
        n447 = call <vilib>:"NT Write String.vi"("String"=w721, "Name"="Auto Selector") -> ()  [unwired: 9 in, 1 out]
      }
      event "Command Selection": Value Change {
        # "Get the params and show in table"
        n448 = event-data() -> ("NewVal"=w727:i32)  [unwired: 1 in]
        n449 = property on="Command Selection" class="MCListbox (strict)"() -> ("ItemNames"=w725:string[][])  [unwired: 2 in, 2 out]
        n450 = call <vilib>:"WPI_DashboardUpdate Command Params.vi"("NewVal"=w727, "Commands"=w725, "Param Tbl"=w726) -> ()  [unwired: 8 in, 1 out]
      }
      event "Execute Command": Value Change {
        # "Started one, Unique ID holds\nresponse"
        n451 = event-data() -> ()  [unwired: 1 in, 1 out]
        n452 = property on="Command Selection" class="MCListbox (strict)"() -> ("ItemNames"=w738:string[][])  [unwired: 2 in, 2 out]
        n453 = Index Array(array=w738, index (row)="Command Selection", index (col)=0) -> (element=w736:string)
        n454 = call <vilib>:"Invoke Commands.vi"("Command Params"="Command Params", "Function Name"=w736) -> ("Params"=w732:u8, "Started"=w731:bool)  [unwired: 7 in, 1 out]
        n455 = Array Subset(array="Command Params", length (row)=w732) -> (w733:string[][])  [unwired: 3 in]
        n456 = Select(t="Executing" ("Cmd Status"), s=w731, f="" ("Cmd Status")) -> (s? t:f=→"Cmd Status":string)
      }
      event "Command Selection": Double Click {
        n457 = event-data() -> ("Row"=w746:i32)  [unwired: 1 in]
        n458 = property on="Command Selection" class="MCListbox (strict)"() -> ("ItemNames"=w749:string[][])  [unwired: 2 in, 2 out]
        n459 = local read "Command Params"() -> (w745:string[][])
        n460 = Index Array(array=w749, index (row)=w746, index (col)=0) -> (element=w747:string)
        n461 = call <vilib>:"Invoke Commands.vi"("Command Params"=w745, "Function Name"=w747) -> ("Params"=w744:u8, "Started"=w739:bool)  [unwired: 7 in, 1 out]
        n462 = Array Subset(array=w745, length (row)=w744) -> (w743:string[][])  [unwired: 3 in]
        n463 = Select(t="Executing" ("Cmd Status"), s=w739, f="" ("Cmd Status")) -> (s? t:f=w740:string)
        n464 = local write "Cmd Status"(w740) -> ()
      }
      event "CheckList": Double Click {
        # "Shift clears all"
        # "Update symbols on the listbox"
        n465 = event-data() -> ("PlatMods.Shift"=w751:bool, "Row"=w753:i32)  [unwired: 1 in]
        n466 = case shown="True" w751 {
          tunnel: w753 -> [w757 _]
          tunnel: 1 -> [w756 _]
          frame False {
            n467 = property on="CheckList" class="LstBox (strict)"() -> ("Item Symbols"=w755:i32[])  [unwired: 2 in, 2 out]
            n468 = Replace Array Subset(array=w755, new element=w756, index=w757) -> (w754:i32[])
            n469 = property on="CheckList" class="LstBox (strict)"("Item Symbols"=w754) -> ()  [unwired: 2 in, 2 out]
          }
          frame True {
            w758 = 0 ("Top Row")
            n470 = property on="CheckList" class="LstBox (strict)"() -> ("Number of Rows"=w760:u32)  [unwired: 2 in, 2 out]
            n471 = Initialize Array(0, w760) -> (w759:i32[])
            n472 = property on="CheckList" class="LstBox (strict)"("Top Row"=w758, "Value"=w758, "Item Symbols"=w759) -> ()  [unwired: 2 in, 2 out]
          }
        }
      }
      event "CheckList": Key Down {
        # "Update symbols on the listbox\nLeft and right keys check and uncheck"
        n473 = event-data() -> ("VKey"=w764:T19)  [unwired: 1 in]
        n474 = case shown="\"Left\", \"Right\"" w764 {
          selector: w764 -> [w769 _]
          tunnel: eventvkey."Left" ("VKey") -> [w767 _]
          frame "Left", "Right" {
            n475 = Equal?(x=w767, y=w769) -> (x = y?=w768:bool)
            n476 = Select(t=0, s=w768, f=1) -> (s? t:f=w770:i32)
            n477 = property on="CheckList" class="LstBox (strict)"() -> ("Item Symbols"=w773:i32[])  [unwired: 2 in, 2 out]
            n478 = Replace Array Subset(array=w773, new element=w770, index="CheckList") -> (w772:i32[])
            n479 = property on="CheckList" class="LstBox (strict)"("Item Symbols"=w772) -> ()  [unwired: 2 in, 2 out]
          }
          frame Default {
          }
        }
      }
      event "Motor.Enable": Value Change {
        # "When the test mode otor enable helper is set, update that\ntree row item's value"
        n480 = event-data() -> ("NewVal"=w779:bool)  [unwired: 1 in]
        n481 = Unbundle("Motor") -> ("Value"=w778:dbl)  [unwired: 1 out]
        n482 = Select(t=w778, s=w779, f=0.0) -> (s? t:f=w776:dbl)
        n483 = call <vilib>:"NT Write Number.vi"("Numeric"=w776, "Name"=w775) -> ()  [unwired: 9 in, 1 out]
      }
      event "Test Slider": Value Change {
        # "When the test mode slider helper is set, update that\ntree row item's value"
        n484 = event-data() -> ("NewVal"=w782:dbl)  [unwired: 1 in]
        n485 = call <vilib>:"NT Write Number.vi"("Numeric"=w782, "Name"=w783) -> ()  [unwired: 9 in, 1 out]
      }
      event "On/Off": Value Change {
        # "When the test mode on/off helper value is set, update that\ntree row item's value"
        n486 = event-data() -> ("NewVal"=w787:bool)  [unwired: 1 in]
        n487 = Boolean To (0,1)(Boolean=w787) -> (0, 1=w786:i16)
        n488 = call <vilib>:"NT Write Number.vi"("Numeric"=w786, "Name"=w785) -> ()  [unwired: 9 in, 1 out]
      }
      event "Rev/Fwd": Value Change {
        # "When the test mode helper value for relays is set, update that\ntree row item's value"
        n489 = event-data() -> ("NewVal.Forward"=w795:bool, "NewVal.Reverse"=w794:bool)  [unwired: 1 in]
        n490 = Boolean To (0,1)(Boolean=w795) -> (0, 1=w791:i16)
        n491 = Boolean To (0,1)(Boolean=w794) -> (0, 1=w793:i16)
        n492 = Negate(x=w793) -> (-x=w792:i16)
        n493 = Add(x=w791, y=w792) -> (x+y=w790:i16)
        n494 = call <vilib>:"NT Write Number.vi"("Numeric"=w790, "Name"=w789) -> ()  [unwired: 9 in, 1 out]
      }
      event "Test Ring": Value Change {
        # "When a test mode helper value is selected from the ring,\nset the tree item's variable to the string value"
        n495 = event-data() -> ("NewVal"=w799:u16)  [unwired: 1 in]
        n496 = property on="Test Ring" class="Ring (strict)"() -> ("Strings []"=w800:string[])  [unwired: 2 in, 2 out]
        n497 = Index Array(array=w800, index=w799) -> (element=w798:string)
        n498 = call <vilib>:"NT Write String.vi"("String"=w798, "Name"=w797) -> ()  [unwired: 9 in, 1 out]
      }
      event "Rec Mode": Value Change {
        # "Update globals for recording mode and path to read log from.\nClear when logging and let NetworkTables set path for vision to\nuse."
        n499 = event-data() -> ("NewVal"=w809:enum32{"Stop", "Record", "Playback"})  [unwired: 1 in]
        n500 = global write "WPI_DashboardLogging Global.vi" "Logging Filename"(path "") -> ()
        n501 = global write "WPI_DashboardLogging Global.vi" "Recording"(w809) -> ()
        n502 = case shown="\"Playback\"" w809 {
          tunnel: w808 -> [_ w811 w820]
          tunnel: [_ _ w819] -> w806
          tunnel: [_ _ w818] -> _
          tunnel: w804 -> [_ _ w816]
          tunnel: cluster{i32, i32} {-250, 170} -> [_ _ w815]
          tunnel: [_ _ T20 {"Image Size"=TRUE, "Image Type"=TRUE, "Pixel Value"=TRUE, "ROI Information"=TRUE, "Zoom Factor"=FALSE} ("Image Information Shown:All Elements")] -> _
          tunnel: [_ _ TRUE ("Zoom Factor")] -> _
          tunnel: w802 -> [_ _ w812]
          frame Default {
          }
          frame "Stop", "Record" {
            # "Place Window too"
            n503 = invoke class="VI" method="FP.Close"(reference=w811) -> (reference out=w810:refnum<vi>)  [unwired: 2 in, 2 out]
            n504 = invoke class="VI" method="Abort VI"(reference=w810) -> ()  [unwired: 2 in, 3 out]
          }
          frame "Playback" {
            n505 = call "Open Playback Panel.vi"("Offset"=w815, "DB VI Ref"=w816, "Playback in"=w820) -> ("Playback out"=w817:refnum<vi>)  [unwired: 8 in]
            n506 = register-events(w817, w812) -> (reference out=w819:refnum<event-registration>, error out=w818:errorcluster)  [unwired: 2 in]
          }
        }
        n507 = call <vilib>:"WPI_DashboardNT Log FieldName Cache.vi"("Operation"=enum16{"Lookup/Add", "Index", "Clear"}."Clear") -> ()  [unwired: 8 in, 3 out]
      }
      event Panel Close {
        w822 = enum32{"Stop", "Record", "Playback"}."Stop" ("Rec Mode")
        # "Playback window has been closed, abort"
        n508 = event-data() -> ()  [unwired: 1 in, 4 out]
        n509 = local write "Rec Mode"(w822) -> ()
        n510 = global write "WPI_DashboardLogging Global.vi" "Recording"(w822) -> ()
      }
      event Panel Close {
        # "Abort playback window and ourself"
        n511 = event-data() -> ()  [unwired: 1 in, 4 out]
        n512 = invoke class="VI" method="FP.Close"(reference=w826) -> (reference out=w825:refnum<vi>)  [unwired: 2 in, 2 out]
        n513 = invoke class="VI" method="Abort VI"(reference=w825) -> (error out=w824:errorcluster)  [unwired: 2 in, 2 out]
        n514 = invoke class="VI" method="Abort VI"(error in=w824) -> ()  [unwired: 2 in, 3 out]
      }
      event User Event {
        n515 = event-data() -> ("IDs"=w833:cluster{"RPC field ID":u16, "Unique ID":u16}, "String"=w832:string)  [unwired: 1 in]
        n516 = Bundle("IDs"=w833, "String"=w832) -> (w831:T9)  [unwired: 1 in]
        n517 = call <vilib>:"Retrieve RPC Response.vi"("RPC Response"=w831) -> ("Output"=w829:string[][])  [unwired: 10 in]
        n518 = Build Array (concatenate)(w827, w829) -> (w828:string[][])
        n519 = local write "Command Params"(w828) -> ()
        n520 = local write "Cmd Status"("" ("Cmd Status")) -> ()
      }
      event "Tree": Double Click {
        n521 = event-data() -> ("PlatMods"=w839:T23, "Tag"=w836:string)  [unwired: 1 in]
        n522 = Unbundle(w839) -> ("Shift"=w838:bool)  [unwired: 4 out]
        n523 = String Subset(string=w836, length (rest)=1 ("length (rest)")) -> (substring=w835:string)  [unwired: 1 in]
        n524 = Not(x=w838) -> (.not. x?=w837:bool)
        n525 = case shown="\"/\"" w835 {
          tunnel: w836 -> [_ w842]
          tunnel: w837 -> [_ w841]
          frame Default {
          }
          frame "/" {
            n526 = call <vilib>:"NT Update Persistence.vi"("Persistence"=w841, "Name"=w842) -> ()  [unwired: 9 in, 1 out]
          }
        }
      }
    }
  }
  n527 = while {
    tunnel: u16 1741 ("timeout ms (25000)") -> [w844]
    stop <- FALSE stop-if-true
    n528 = TCP Create Listener(10:w844) -> (0:w843:errorcluster, 3:w845:refnum<k5>)  [unwired: 4 in, 1 out]
    n529 = case shown="No Error" w843 {
      selector: w843 -> [w847 _]
      tunnel: w845 -> [w848 _]
      frame No Error {
        n530 = while {
          tunnel: w848 -> [w851]
          tunnel: w847 -> [w850]
          stop <- FALSE stop-if-true
          n531 = TCP Wait On Listener(8:w850, 11:w851) -> (0:w852:errorcluster, 4:w853:refnum<k5>)  [unwired: 2 in, 3 out]
          n532 = local write "TCP"(w853) -> ()
          n533 = case shown="No Error" w852 {
            frame No Error {
            }
            frame Error {
              n534 = Wait (ms)(milliseconds to wait=u32 1000) -> ()  [unwired: 1 out]
            }
          }
        }
      }
      frame Error {
        n535 = Wait (ms)(milliseconds to wait=u32 1000) -> ()  [unwired: 1 out]
      }
    }
  }
  n536 = local write "Dashboard Tab"(T1."Checklist" ("Dashboard Tab")) -> ()
  n537 = property on="On/Off" class="Bool (strict)"("Visible"=w19) -> ()  [unwired: 2 in, 2 out]
  n538 = property on="Motor" class="Clust (strict)"("Visible"=w19) -> ()  [unwired: 2 in, 2 out]
  n539 = property on="Progress" class="Clust (strict)"("Visible"=w19) -> ()  [unwired: 2 in, 2 out]
  n540 = property on="Test Ring" class="Ring (strict)"("Visible"=w19) -> ()  [unwired: 2 in, 2 out]
  n541 = property on="Rev/Fwd" class="Clust (strict)"("Visible"=w19) -> ()  [unwired: 2 in, 2 out]
  n542 = local write "Command Selection"(u16 0 ("milliseconds to wait")) -> ()
  n543 = local write "Command Params"(string[][] [] ("Command Params")) -> ()
  n544 = global write "WPI_DashboardLogging Global.vi" "Recording"(w25) -> ()
  n545 = local write "Rec Mode"(w25) -> ()
  n546 = call <vilib>:"NT Write String.vi"("String"="Select Auto", "Name"="Auto Selector") -> ()  [unwired: 9 in, 1 out]
  n547 = while {
    tunnel: w1 -> [_]
    stop <- FALSE stop-if-true
    # "Error Message Handling"
    n548 = local read "Tilt_Safety_Override"() -> (w894:bool)
    n549 = local read "Tilt_Interlock"() -> (w880:bool)
    n550 = local read "Super_Test_Mode"() -> (w896:bool)
    n551 = local read "Elevator_Manual"() -> (w895:bool)
    n552 = local read "Master_Safety_Override_1"() -> (w890:bool)
    n553 = local read "Master_Safety_Override_2"() -> (w891:bool)
    n554 = local read "Check_Limit_Switch"() -> (w886:bool)
    n555 = local read "Elevator_Stall"() -> (w883:bool)
    n556 = local read "E1 Warning"() -> (w877:bool)
    n557 = local read "E2 Warning"() -> (w876:bool)
    n558 = local read "E3 Warning"() -> (w875:bool)
    n559 = local read "State_Conflict"() -> (w868:bool)
    n560 = local read "Battery_Critical"() -> (w865:bool)
    n561 = And(x=w890, y=w891) -> (x .and. y?=w889:bool)
    n562 = Build Array(1000.0, 1000.0, 1000.0 ("element"), 1000.0 ("element"), 10.0 ("element"), 10.0 ("element"), 3.0 ("element"), 10.0 ("element"), 10.0 ("element"), 10.0 ("element"), 3.0 ("element"), 10.0 ("element"), 10.0 ("element")) -> (w898:dbl[])
    n563 = Build Array("super test mode", "elevator in manual mode", "tilt safety disabled" ("element"), "all safeties disabled" ("element"), "elevator limit switch failure" ("element"), "elevator is stalling" ("element"), "reset tilt interlock" ("element"), "elevator motor 1 has failed" ("element"), "elevator motor 2 has failed" ("element"), "elevator motor 3 has failed" ("element"), "eject game piece" ("element"), "battery low" ("element"), "pressure leak detected" ("element")) -> (w901:string[])
    n564 = Build Array(w896, w895, w894, w889, w886, w883, w880, w877, w876, w875, w868, w865, FALSE) -> (w860:bool[])
    n565 = call "ErrorMessageBuilder.vi"("Error Triggers"=w860, "Delays (s)"=w898, "Error Messages"=w901) -> ("Combined Error String"=w858:string)  [unwired: 2 in]
    "Combined Error String" <- w858
    n566 = Not Equal?(x="", y=w858) -> (x != y?=w859:bool)
    n567 = Wait (ms)(milliseconds to wait=u32 200) -> ()  [unwired: 1 out]
    n568 = case shown="True" w859 {
      tunnel: w858 -> [_ w905]
      frame False {
      }
      frame True {
        n569 = call "TextToSpeech.vi"("Text To Be Spoken"=w905) -> ()  [unwired: 9 in, 2 out]
      }
    }
  }
